vi "eyecat MAX v2-1_JS_160308.vi"() -> ()   [LabVIEW 2014]
doc: "This VI is an upgrade from the WIN 1_v4 that implements the ageing subrutine"
uses:
  Buttons/String output.ctl
  <vilib>/Utility/miscctls.llb/LVRowAndColumnTypeDef.ctl
  Buttons/Numeric control.ctl
  Buttons/String input.ctl
  Buttons/Numeric indicator.ctl
  Controls Win/Control 3.ctl
  <vilib>/Platform/TimedLoop/XDataNode/nitl_modes.ctl
  <vilib>/Platform/TimedLoop/XDataNode/timing_clust.ctl
  <vilib>/Platform/TimedLoop/XDataNode/wakeup.ctl
  <vilib>/Utility/file.llb/Write To Spreadsheet File (string).vi
  <vilib>/Utility/file.llb/Read From Spreadsheet File (string).vi
  <vilib>/Utility/file.llb/Read From Spreadsheet File (DBL).vi
  <vilib>/regexp/Match Regular Expression.xnode
  <vilib>/Platform/TimedLoop/XDataNode/XDataNode.xnode
  <vilib>/Platform/TimedLoop/XDataNode/XDNodeRunTimeDep.lvlib
panel:
  out "Mexa_One Emissions":dbl[](array[numeric])
  out "Advanced Logging":bool
  out "Full System":bool
  out "MKS":bool
  in  "Alarm":bool
  in  "Analyser":bool
  in  "MFC":bool
  in  "System":bool
  in  "Ageing":bool
  in  "Performance":bool
  in  "Home":bool
  out "NO":dbl[](array[numeric])
  out "CO":dbl[](array[numeric])
  out "Mexa One":bool
  out "Pressure":dbl
  in  "Duration -1":i32
  in  "Demo Sync":i32
  in  "Demo On":bool
  in  "FlowGuide":bool
  in  "Mean(Off)/Interval(On) 2":bool
  in  "Flow Band %":dbl=1.04
  in  "Flow Sync":i32
  out "Emissions":dbl[](array[numeric])
  in  "Temperature Sync":i32
  in  "TempGuide":bool
  in  "Temp Band %":dbl=1.04
  in  "Mean(Off)/Interval(On)":bool
  in  "MKS 5Hz":bool
  out "output cluster":T2
  out "Lambda":dbl[](array[numeric])
  out "MKS HC":dbl
  in  "HC Index":i32
  out "Open/Closed \nLoop":dbl[](array[numeric])
  out "Air Cyc 2":dbl[](array[numeric])
  in  "Cycle size":i32
  out "ExtAnDn":bool
  out "ExtAnUp":bool
  out "HC Cyc 2":dbl[](array[numeric])
  out "SO Valve 2":dbl[](array[numeric])
  out "SO Valve 1":dbl[](array[numeric])
  out "Air Bal":dbl[](array[numeric])
  out "HC Bal":dbl[](array[numeric])
  out "Air Cyc 1":dbl[](array[numeric])
  out "HC Cyc 1":dbl[](array[numeric])
  out "File name":string
  out "Log?":bool
  out "Connected":bool
  out "Furnace temp 2":dbl
  out "Log interval (seconds)":T1
  in  "Flow rate Age":dbl
  in  "Inlet temp Age":dbl
  out "Stopped?":bool
  in  "Stop Cmd":T1
  out "Connected?":bool
  out "Error":dbl
  out "Iteration Duration":i64
  out "Finished Late? [i-1]":bool
  out "Furnace temp 1":dbl
  out "stop 2":bool
  in  "Enum 1":i16=1
  in  "Acknowledge":bool
  out "Test number":u16
  out "Flag1":bool=TRUE
  out "EditPos Subc":T3
  out "Flag 2":bool=TRUE
  in  "Tab Control":T4(tab)
  out "Warm Up":bool
  in  "Leak Test":bool
  in  "Stop Test":bool
  in  "Log Test Data":bool
  in  "Start Test":bool
  in  "Adv Settings":bool
  out "Doors Unlocked":bool
  in  "Temperature Limit (°C)":T1=1200.0 min=0.0 max=1200.0 step=1.0
  in  "File Name":T5="Test"
  in  "File Path":path=path "C:/DATA LOG"
  out "Fail":bool
  out "Pass":bool
  in  "Select Test Type":T6(radio)
  out "Standby":bool
  out "Doors Open":bool
  out "Extractor Fan On":bool
  out "Test In Progress":bool
  out "Cool Down":bool
  out "System Alarm":bool
  in  "Inlet Temperature (°C)":T1=400.0 min=350.0 max=1000.0 step=1.0
  in  "Inlet LAMBDA Lean":T1=1.2 min=1.02 max=3.0 step=0.001
  in  "Test Stop temperature (°C)":T1=300.0 min=100.0 max=1000.0 step=1.0
  in  "Test Start Temperature (°C)":T1=125.0 min=0.0 max=500.0 step=1.0
  in  "Furnace Ramp Rate (°C/min)":T1=15.0 min=1.0 max=50.0 step=0.1
  in  "NO:CO Ratio":T1=1.1 min=1.0 max=5.0 step=0.1
  in  "Inlet O2 (%)":T1=0.5 min=0.0 max=14.0 step=0.01
  in  "Inlet LAMBDA":T1=1.0 min=0.6 max=3.0 step=0.001
  out "Space Velocity (h-1)":T7
  out "Vol Flow @ STP (l/min)":T7
  in  "Test Flow Rate(g/s)":T1 min=0.0 max=100.0 step=0.01
  out "Sample Volume (litres)":T7
  in  "Number of Samples":T1=1.0 min=1.0 max=6.0 step=1.0
  in  "Sample Diameter (mm)":T1
  out "CO Theory (%) NO":T7 format="%#_3g"
  out "CO Theory (%)":T7 format="%#_3g"
  out "HC Theory (%)":T7
  in  "Sample Length (mm)":T1 min=0.0 step=0.5
  in  "NO ppm SW":dbl=500.0 caption="NO (ppm)" min=0.0 max=500.0 step=1.0
  in  "NO ppm Loff":T1 caption="NO ppm"
  in  "Delete sCycle":bool
  in  "Load sCycle":bool
  in  "Save sCycle":bool
  in  "Clear subcycle":bool
  in  "Clear Cycle Pattern":bool
  in  "Save Cycle":bool
  in  "Load Cycle":bool
  in  "Delete Cycle":bool
  out "Test Compiled":bool
  in  "Compile Test Button":bool
  in  "Sub-Cycle List":i32(listbox)=1
  in  "Cycle List":i32(listbox)=2
  out "Total Test Duration (hrs)":T8
  in  "Ageing Gas":enum32{"Radio Selection 1", "Radio Selection 2"}(radio)
  in  "Sub-Cycle Pattern":string[][](table) caption="Subcycle pattern"
  in  "Total Number of Cycles":T1=1.0 min=1.0 max=10000.0 step=1.0
  in  "Cycle Pattern":string[][](table)
  in  "Sub-Cycle Name":T5
  in  "Cycle Name":T5
  out "Heat Exchanger Temperatures (°C)":dynamicdata(graph)
  out "Flow Rate (g/s)":dynamicdata(graph)
  out "Sample Temperatures (°C)":dynamicdata(graph)
  out "System Temperatures (°C)":dynamicdata(graph)
  in  "Graph 1 Box":string(combo)="CO"
  in  "Graph 4 Box":string(combo)="NO"
  in  "Graph 3 Box":string(combo)="Air Cycle 1"
  in  "Graph 2 Box":string(combo)="HC Cycle 1"
  out "MFC Graph 4":dynamicdata(graph)
  out "MFC Graph 3":dynamicdata(graph)
  out "MFC Graph 1":dynamicdata(graph)
  out "MFC Graph 2":dynamicdata(graph)
  out "HC Concentration (ppm)":dynamicdata(graph)
  out "Lambda":dynamicdata(graph)
  out "O2/CO Concentration":dynamicdata(graph)
  out "NO Concentration (ppm)":dynamicdata(graph)
  in  "Purge System":bool
  in  "Alarm ack":bool
  in  "Clear log":bool
  out "Table":string[][](table)
  out "Soft Alarm":bool
  out "Hard Alarm":bool
  # "1% = 0.01"
  # "Test Type"
  # "Test Commands"
  # "System Indicators"
  # "Leak Test"
  # "Catalyst Specification"
  # "Lightoff Settings"
  # "Furnace Lightoff Settings"
  # "Sweep Settings"
  # "CO/HC Lightoff Settings"
  # "0.96 < lambda < 0.85"
  # "1.02< lambda < 1.6"
  # "350 < Tinlet < 1000"
  # "NO Lightoff Settings"
  # "Flow Specification"
  # "Cycle Compiled"
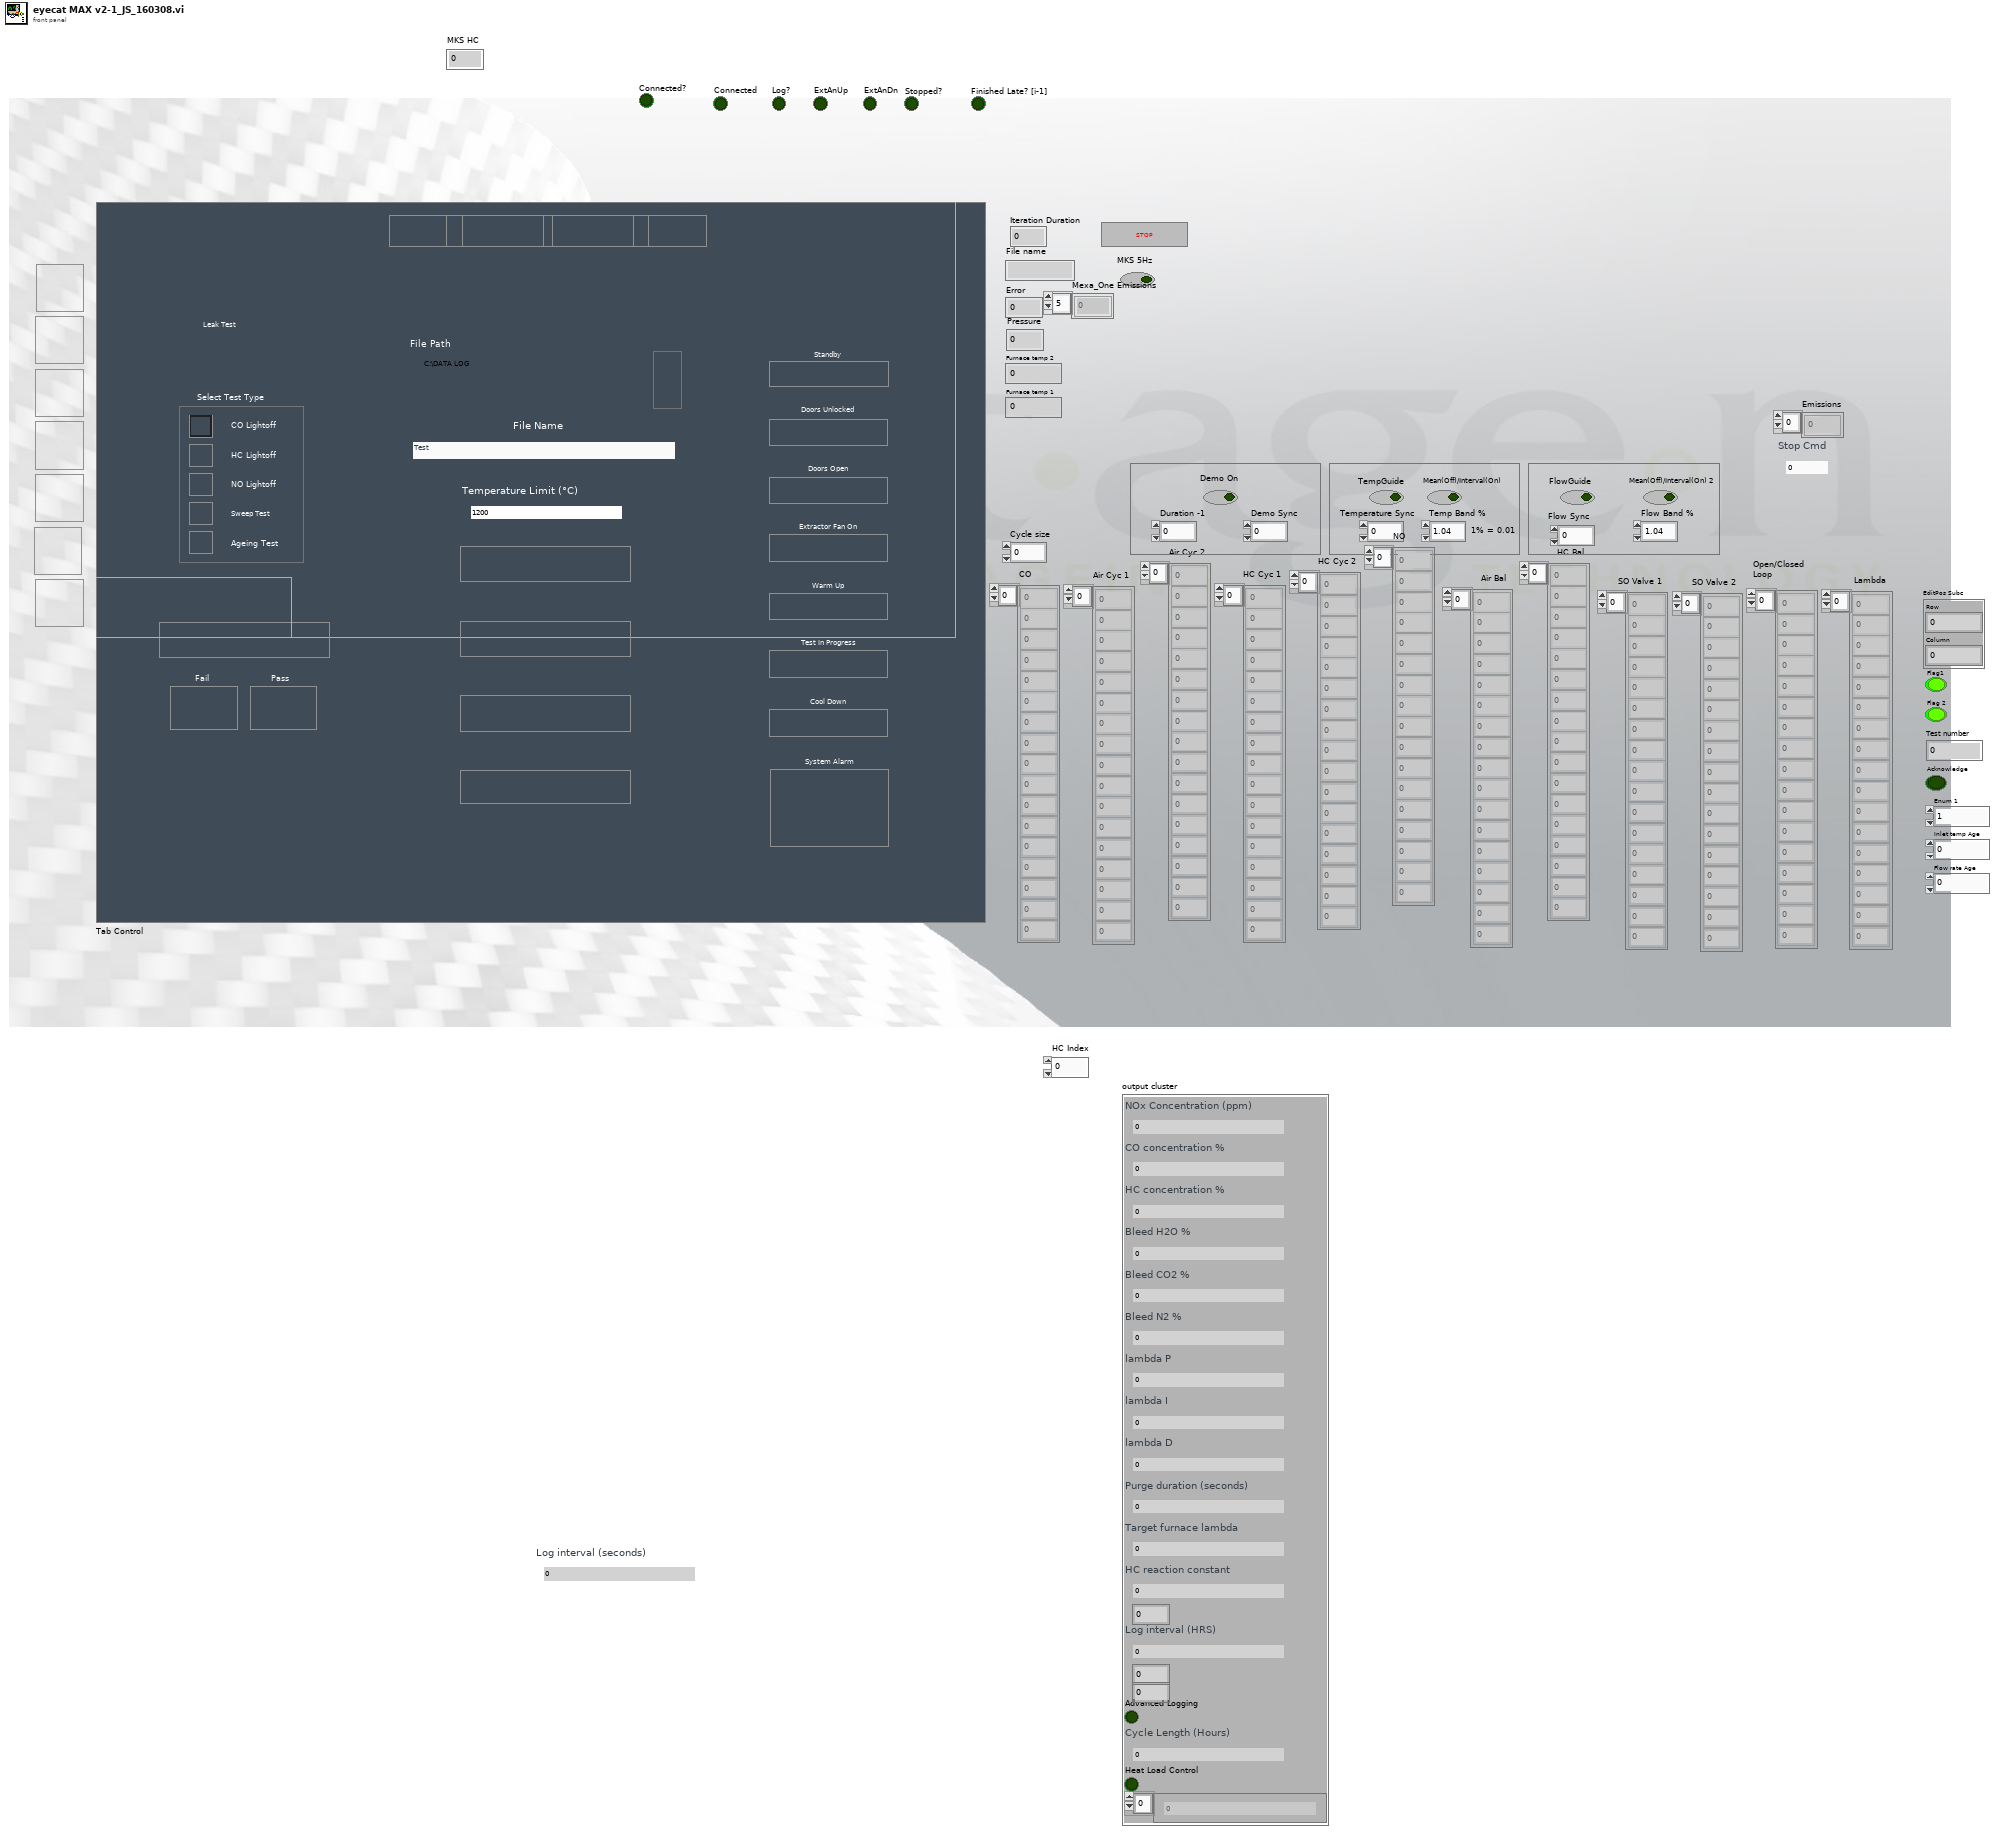
[diagram p1: front panel]
types:
  T1 = typedef "Numeric control.ctl" = dbl
  T2 = cluster{"NOx Concentration (ppm)":T1, "CO concentration %":T1, "HC concentration %":T1, "Bleed H2O %":T1, "Bleed CO2 %":T1, "Bleed N2 %":T1, "lambda P":T1, "lambda I":T1, "lambda D":T1, "Purge duration (seconds)":T1, "Target furnace lambda":T1, "HC reaction constant":T1, i16, "Log interval (HRS)":T1, i16, i16, "Advanced Logging":bool, "Cycle Length (Hours)":T1, "Heat Load Control":bool, T1[]}
  T3 = typedef "LVRowAndColumnTypeDef.ctl" = cluster{"Row":i32, "Column":i32}
  T4 = enum32{"MAIN", "PERFORMANCE TEST SETUP", "AGEING TEST SETUP", "SYSTEM DATA", "MFC", "ANALYSER DATA", "ALARM LOG"}
  T5 = typedef "String input.ctl" = string
  T6 = enum32{"CO Lightoff", "HC Lightoff", "NO Lightoff", "Sweep Test", "Ageing Test"}
  T7 = typedef "Numeric indicator.ctl" = dbl
  T8 = typedef "String output.ctl" = string
  T9 = typedef "XDNodeRunTimeDep.lvlib/nitl_modes.ctl" = enum32{"No Change", "Process missed periods, maintain original phase", "Discard missed periods, maintain original phase", "Process missed periods, ignore original phase", "Discard missed periods, ignore original phase"}
  T10 = typedef "Control 3.ctl" = enum16{"main", "start test", "save subc", "load subc", "delete subc", "clear table 1", "update list 1", "save cycle", "load cycle", "delete cycle", "clear table 2", "update list 2", "calc HC CO", "Total time calc", "update Cycle pattern ", "load cycle name", "convert to num", "load test array", "check scycle name", "check cycle name", "Multigas connect", "Multigas disconnect", "Leak Test", "Import Cycle", "Display Graph"}
  T11 = enum8{"Enabled", "Disabled", "Disabled and Grayed Out"}
  T12 = typedef "XDNodeRunTimeDep.lvlib/timing_clust.ctl" = cluster{"Expected End [f-1]":u64, "Actual End [f-1]":u64, "Finished Late? [f-1]":bool, "Expected End [i-1]":u64, "Actual End [i-1]":u64, "Finished Late? [i-1]":bool, "Expected Start [i]":u64, "Actual Start [i]":u64, "Expected Start [f]":u64, "Actual Start [f]":u64, "Source Name":string, "Structure Name":string, "Period":i64, "Deadline":i64, "Offset":i64, "Start":i64, "Priority":i32, "Timeout":i32, "Mode":T9, "Wakeup Reason":T13, "Error":errorcluster, "Source Type":string, "Secondary Source Type":string, "Global End Time":u64, "Global Start Time":u64, "Frame Duration":u64, "Iteration Duration":u64, "Assigned CPU":i32, "I/O Scan Engine Mode":u32}
  T13 = typedef "XDNodeRunTimeDep.lvlib/wakeup.ctl" = enum32{"Normal", "Aborted", "Asynchronous wakeup", "Timing source error", "Timed loop error", "Timeout"}
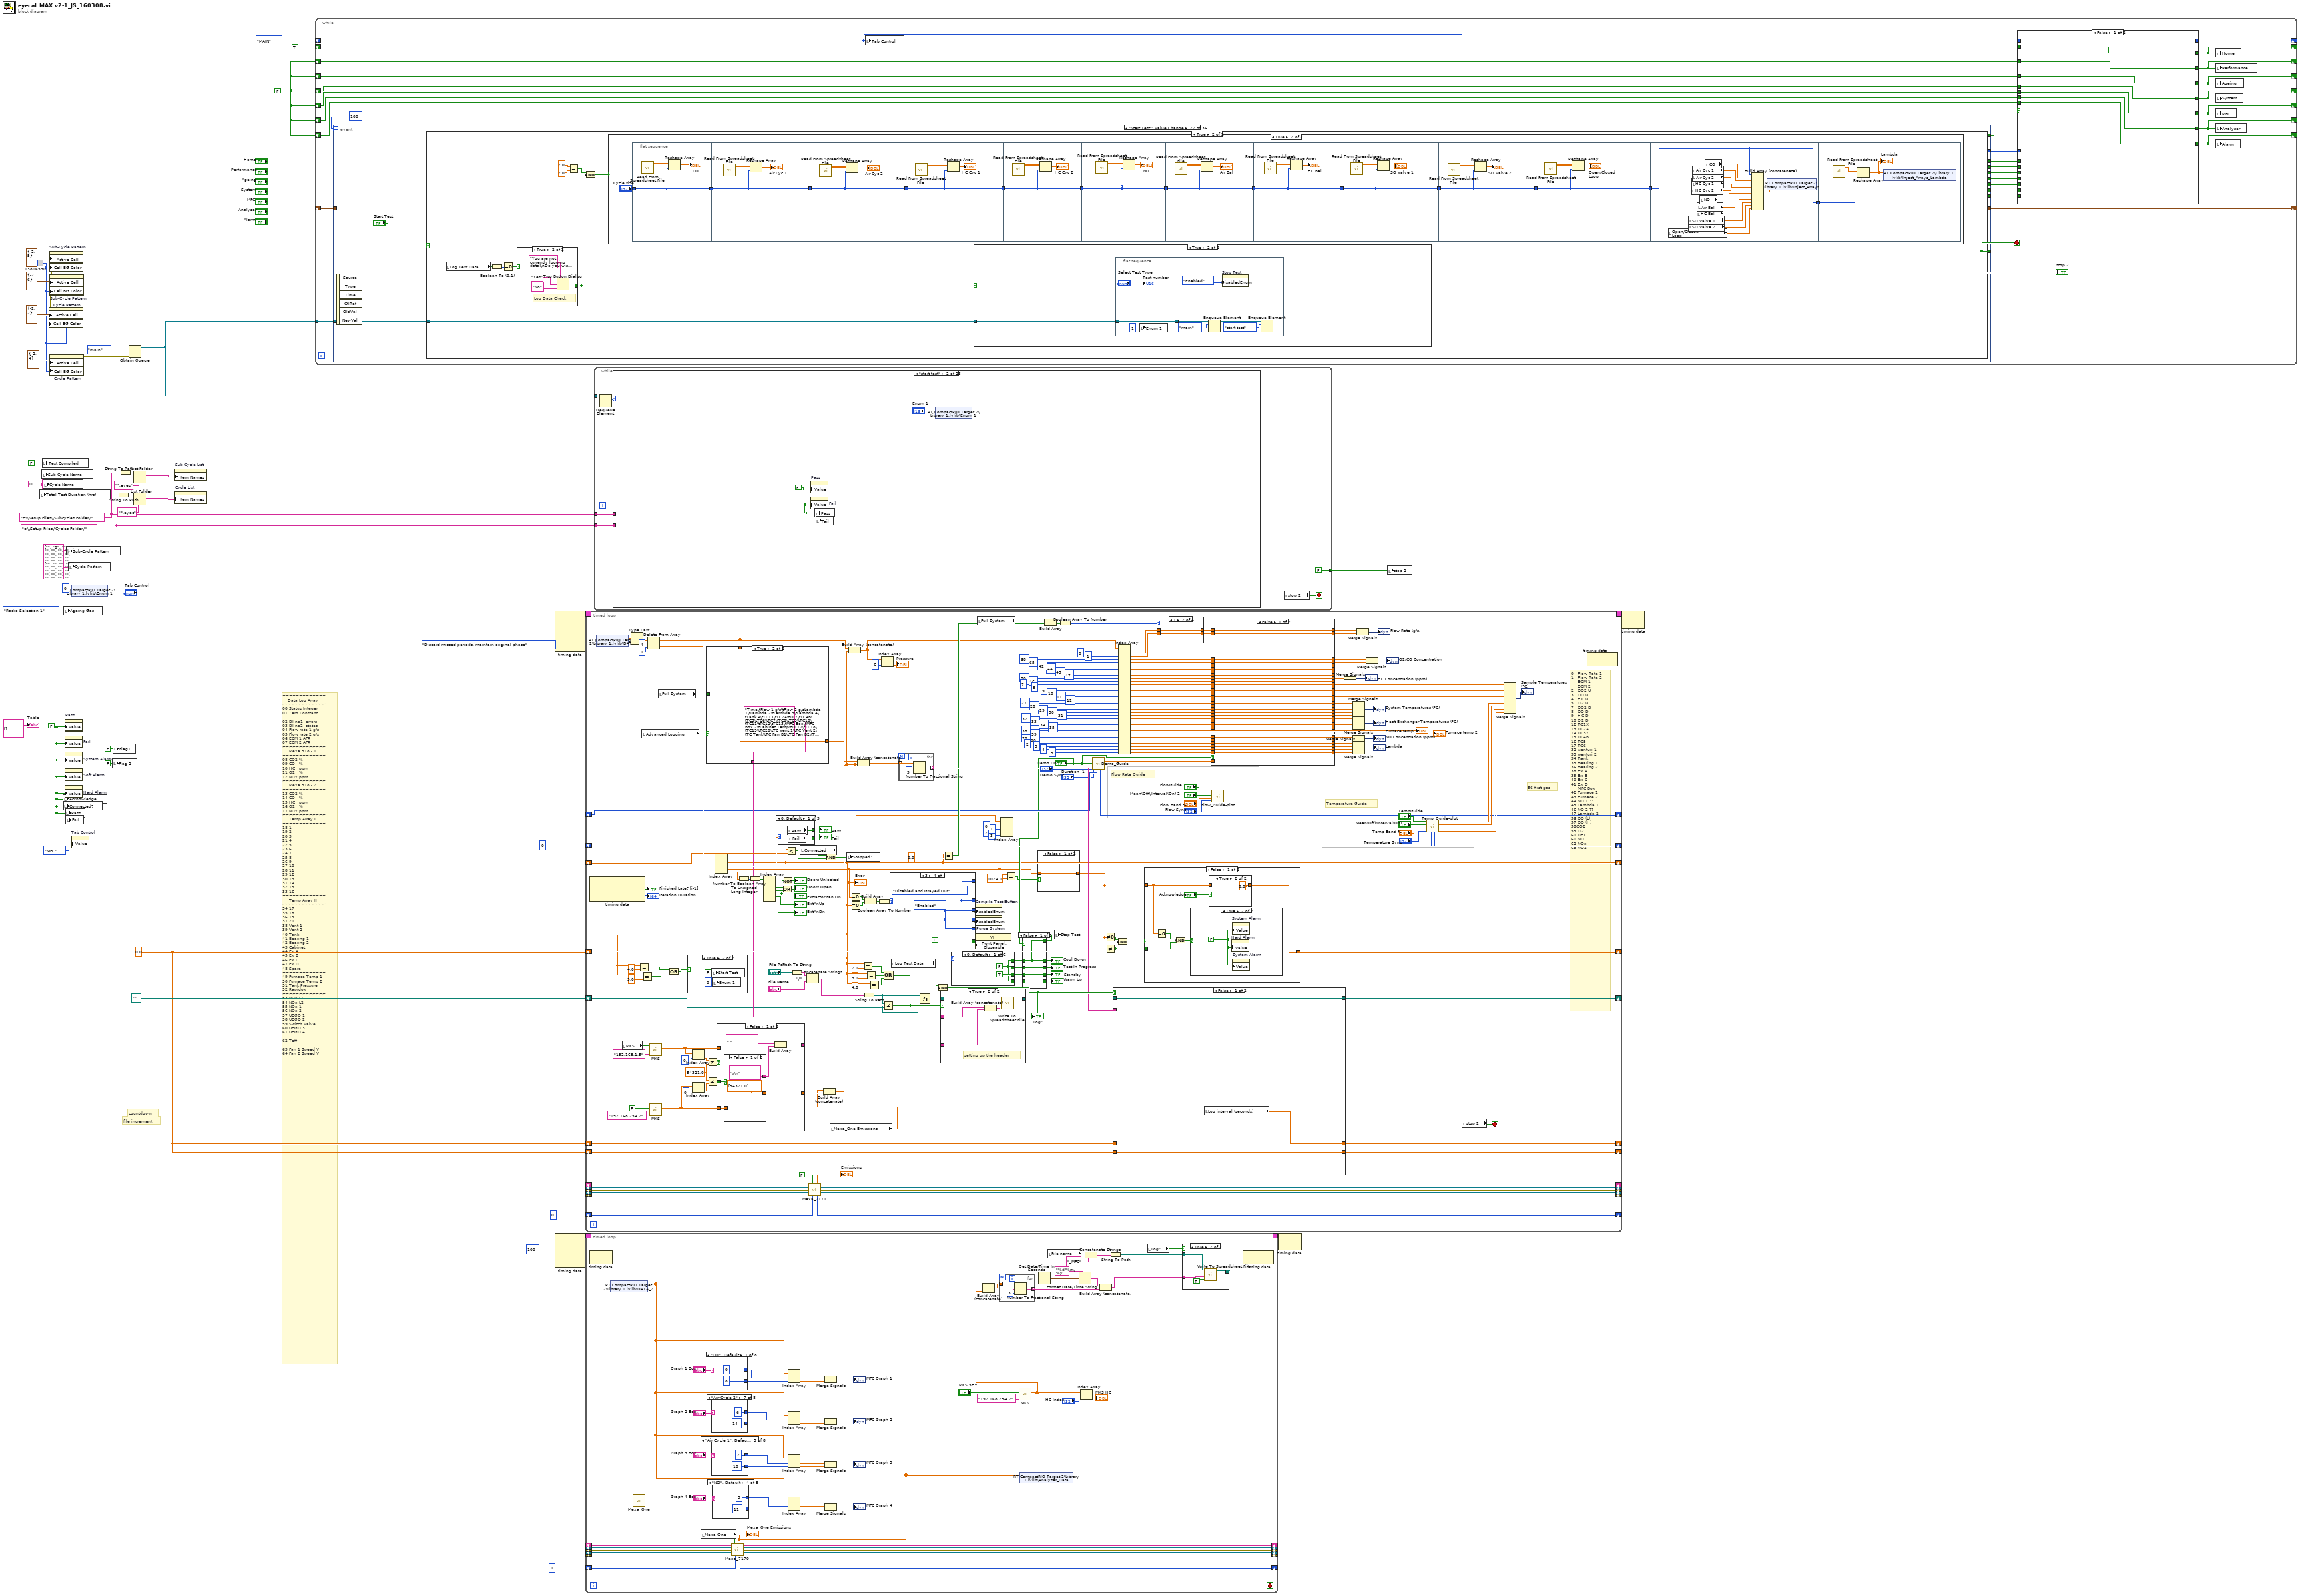
[diagram p0: block diagram]
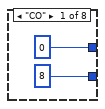
[diagram p2: hidden frame]
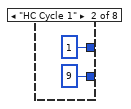
[diagram p3: hidden frame]
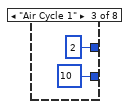
[diagram p4: hidden frame]
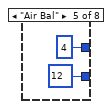
[diagram p5: hidden frame]
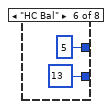
[diagram p6: hidden frame]
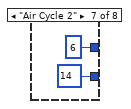
[diagram p7: hidden frame]
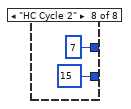
[diagram p8: hidden frame]
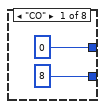
[diagram p9: hidden frame]
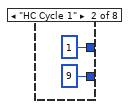
[diagram p10: hidden frame]
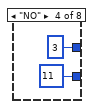
[diagram p11: hidden frame]
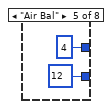
[diagram p12: hidden frame]
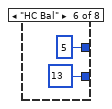
[diagram p13: hidden frame]
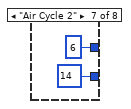
[diagram p14: hidden frame]
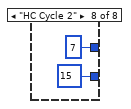
[diagram p15: hidden frame]
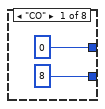
[diagram p16: hidden frame]
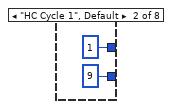
[diagram p17: hidden frame]
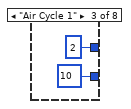
[diagram p18: hidden frame]
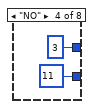
[diagram p19: hidden frame]
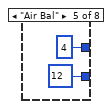
[diagram p20: hidden frame]
diagram:
  (unwired) 0 ("index")
  w2 = FALSE
  (unwired) 0 ("index")
  w10 = FALSE
  w9 = 0.0 ("y")
  w25 = ""
  w28 = "c:\\Setup Files\\Cycles Folder\\"
  w34 = u32 13816530
  w26 = "c:\\Setup Files\\Subcycles Folder\\"
  # "~~~~~~~~~~~~~\n    Data Log Array\n~~~~~~~~~~~~~\n00 Status Integer\n01 Zero Constant\n\n02 DI no1 -errors\n03 DI no2 -states\n04 Flow rate 1 g/s\n05 Flow rate 2 g/s\n06 ECM 1 AFR\n07 ECM 2 AFR\n~~~~~~~~~~~~~\n     Mexa 518 - 1\n~~~~~~~~~~~~~\n08 CO2 %\n09 CO   %\n10 HC   ppm\n11 O2   %\n12 NOx ppm\n~~~~~~~~~~~~~\n     Mexa 518 - 2\n~~~~~~~~~~~~~\n13 CO2 %\n14 CO   %\n15 HC   ppm\n16 O2   %\n17 NOx ppm\n~~~~~~~~~~~~~\n     Temp Array I\n~~~~~~~~~~~~~\n18 1\n19 2 \n20 3\n21 4\n22 5\n23 6\n24 7\n25 8\n26 9\n27 10\n28 11\n29 12\n30 13\n31 14\n32 15\n33 16\n~~~~~~~~~~~~~\n     Temp Array II\n~~~~~~~~~~~~~\n34 17\n35 18\n36 19\n37 20\n38 Vent 1\n39 Vent 2\n40 Tank\n41 Bearing 1\n42 Bearing 2\n43 Cabinet\n44 Ex A\n45 Ex B\n46 Ex C\n47 Ex D\n48 Spare\n~~~~~~~~~~~~~\n49 Furnace Temp 1\n50 Furnace Temp 2\n51 Tank Pressure\n52 Rapidox\n~~~~~~~~~~~~~\n53 NOx L1\n54 NOx L2\n55 NOx 1\n56 NOx 2\n57 UEGO 1\n58 UEGO 2\n59 Switch Valve\n60 UEGO 3\n61 UEGO 4\n\n62 Teff\n\n63 Fan 1 Speed V\n64 Fan 2 Speed V"
  # "file increment"
  # "countdown"
  n1 = local write "Total Test Duration (hrs)"(w25) -> ()
  n2 = local write "Sub-Cycle Name"(w25) -> ()
  n3 = local write "Test Compiled"(FALSE ("Cycle Compiled")) -> ()
  n4 = local write "Cycle Name"(w25) -> ()
  n5 = property on="Sub-Cycle Pattern" class="Tbl (strict)"("Active Cell"=T3 {"Row"=-2, "Column"=5} ("Active Cell:Active Cell"), "Cell BG Color"=w34) -> (error out=w39:errorcluster)  [unwired: 2 in, 1 out]
  n6 = property on="Sub-Cycle Pattern" class="Tbl (strict)"(error in=w39, "Active Cell"=T3 {"Row"=-2, "Column"=6} ("Active Cell:Active Cell"), "Cell BG Color"=w34) -> (error out=w38:errorcluster)  [unwired: 1 in, 1 out]
  n7 = property on="Cycle Pattern" class="Tbl (strict)"(error in=w38, "Active Cell"=T3 {"Row"=-2, "Column"=2} ("Active Cell:Active Cell"), "Cell BG Color"=w34) -> (error out=w36:errorcluster)  [unwired: 1 in, 1 out]
  n8 = property on="Cycle Pattern" class="Tbl (strict)"(error in=w36, "Active Cell"=T3 {"Row"=-2, "Column"=4} ("Active Cell:Active Cell"), "Cell BG Color"=w34) -> (error out=w33:errorcluster)  [unwired: 1 in, 1 out]
  n9 = local write "Acknowledge"(w10) -> ()
  n10 = local write "Connected?"(w10) -> ()
  n11 = local write "Ageing Gas"(enum32{"Radio Selection 1", "Radio Selection 2"}."Radio Selection 1" ("Ageing Gas")) -> ()
  n12 = property on="Pass" class="Bool (strict)"("Value"=w10) -> ()  [unwired: 2 in, 2 out]
  n13 = property on="Fail" class="Bool (strict)"("Value"=w10) -> ()  [unwired: 2 in, 2 out]
  n14 = property on="System Alarm" class="Bool (strict)"("Value"=w10) -> ()  [unwired: 2 in, 2 out]
  n15 = property on="Soft Alarm" class="Bool (strict)"("Value"=w10) -> ()  [unwired: 2 in, 2 out]
  n16 = property on="Hard Alarm" class="Bool (strict)"("Value"=w10) -> ()  [unwired: 2 in, 2 out]
  n17 = local write "Pass"(w10) -> ()
  n18 = local write "Fail"(w10) -> ()
  n19 = local write "Sub-Cycle Pattern"(string[][] [["", "0", "", "", "", "", "", "", "", "", "", "", ""], ["", "", "", "", "", "", "", "", "", "", "", "", ""], ["", "", "", "", "", "", "", "", "", "", "", "", ""], ["", "", "", "", "", "", "", "", "", "", "", "", ""], ["", "", "", "", "", "", "", "", "", "", "", "", ""], ["", "", "", "", "", "", "", "", "", "", "", "", ""], ["", "", "", "", "", "", "", "", "", "", "", "", ""], ["", "", "", "", "", "", "", "", "", "", "", "", ""], ["", "", "", "", "", "", "", "", "", "", "", "", ""], ["", "", "", "", "", "", "", "", "", "", "", "", ""], ["", "", "", "", "", "", "", "", "", "", "", "", ""], ["", "", "", "", "", "", "", "", "", "", "", "", ""], ["", "", "", "", "", "", "", "", "", "", "", "", ""], ["", "", "", "", "", "", "", "", "", "", "", "", ""], ["", "", "", "", "", "", "", "", "", "", "", "", ""], ["", "", "", "", "", "", "", "", "", "", "", "", ""], ["", "", "", "", "", "", "", "", "", "", "", "", ""], ["", "", "", "", "", "", "", "", "", "", "", "", ""], ["", "", "", "", "", "", "", "", "", "", "", "", ""], ["", "", "", "", "", "", "", "", "", "", "", "", ""], ["", "", "", "", "", "", "", "", "", "", "", "", ""], ["", "", "", "", "", "", "", "", "", "", "", "", ""], ["", "", "", "", "", "", "", "", "", "", "", "", ""], ["", "", "", "", "", "", "", "", "", "", "", "", ""], ["", "", "", "", "", "", "", "", "", "", "", "", ""], ["", "", "", "", "", "", "", "", "", "", "", "", ""], ["", "", "", "", "", "", "", "", "", "", "", "", ""], ["", "", "", "", "", "", "", "", "", "", "", "", ""], ["", "", "", "", "", "", "", "", "", "", "", "", ""], ["", "", "", "", "", "", "", "", "", "", "", "", ""], ["", "", "", "", "", "", "", "", "", "", "", "", ""]]) -> ()
  n20 = local write "Cycle Pattern"(string[][] [["", "", "", "", ""], ["", "", "", "", ""], ["", "", "", "", ""], ["", "", "", "", ""], ["", "", "", "", ""], ["", "", "", "", ""], ["", "", "", "", ""], ["", "", "", "", ""], ["", "", "", "", ""], ["", "", "", "", ""], ["", "", "", "", ""], ["", "", "", "", ""], ["", "", "", "", ""], ["", "", "", "", ""], ["", "", "", "", ""], ["", "", "", "", ""], ["", "", "", "", ""], ["", "", "", "", ""], ["", "", "", "", ""], ["", "", "", "", ""], ["", "", "", "", ""], ["", "", "", "", ""], ["", "", "", "", ""], ["", "", "", "", ""], ["", "", "", "", ""], ["", "", "", "", ""], ["", "", "", "", ""], ["", "", "", "", ""], ["", "", "", "", ""], ["", "", "", "", ""], ["", "", "", "", ""]]) -> ()
  n21 = shared-variable "RT CompactRIO Target 2\\Library 1.lvlib\\Enum 1"(u16 0 ("Enum 1")) -> ()  [unwired: 1 in, 1 out]
  n22 = property on="Tab Control" class="TabCtl (strict)"("Value"=T4."MFC" ("Tab Control")) -> ()  [unwired: 2 in, 2 out]
  n23 = local write "Flag 2"(FALSE) -> ()
  n24 = local write "Flag1"(FALSE) -> ()
  n25 = String To Path(string=w28) -> (path=w29:path)
  n26 = String To Path(string=w26) -> (path=w31:path)
  n27 = Obtain Queue(element data type=Control_3."main" ("Enum"), error in (no error)=w33) -> (queue out=w42:refnum<queue>)  [unwired: 3 in, 2 out]
  n28 = List Folder(path=w29, pattern="*.eyec") -> (filenames=w30:string[])  [unwired: 2 in, 3 out]
  n29 = List Folder(path=w31, pattern="*.eyes") -> (filenames=w32:string[])  [unwired: 2 in, 3 out]
  n30 = property on="Sub-Cycle List" class="LstBox (strict)"("Item Names"=w32) -> ()  [unwired: 2 in, 2 out]
  n31 = property on="Cycle List" class="LstBox (strict)"("Item Names"=w30) -> ()  [unwired: 2 in, 2 out]
  n32 = while {
    tunnel: w42 -> [w73]
    shift-right: [w71] -> _
    shift-left: _ -> [w70]
    shift-right: [w68] -> _
    shift-left: T4."MAIN" ("Tab Control") -> [w67]
    shift-right: [w56] -> _
    shift-left: w2 -> [w49]
    shift-right: [w57] -> _
    shift-left: TRUE -> [w50]
    shift-right: [w55] -> _
    shift-left: w2 -> [w44]
    shift-right: [w54] -> _
    shift-left: w2 -> [w45]
    shift-right: [w53] -> _
    shift-left: w2 -> [w46]
    shift-right: [w52] -> _
    shift-left: w2 -> [w47]
    shift-right: [w51] -> _
    shift-left: w2 -> [w48]
    stop <- w69 stop-if-true
    n33 = event shown="[21] \"Start Test\": Value Change" {
      selector: _ -> [_ _ _ _ _ _ _ _ _ _ _ _ _ _ _ _ _ _ _ _ _ _ _ _ _ _ _ _ _ _ _ _ _ _ _ _]
      dyn-events: _ -> [_ _ _ _ _ _ _ _ _ _ _ _ _ _ _ _ _ _ _ _ _ _ _ _ _ _ _ _ _ _ _ _ _ _ _ _]
      timeout: 100 -> [_ _ _ _ _ _ _ _ _ _ _ _ _ _ _ _ _ _ _ _ _ _ _ _ _ _ _ _ _ _ _ _ _ _ _ _]
      tunnel: w73 -> [w92 w94 _ w103 w111 w118 w125 w136 w140 w151 w156 w159 w164 w186 w194 w195 _ _ _ _ w239 w250 _ w342 w366 _ w380 _ _ _ _ _ _ _ _ _]
      tunnel: [w90 w93 _ w104 w110 w117 w124 w135 w138 w146 w153 w158 w162 w183 _ _ _ _ _ _ _ _ _ _ _ _ _ _ _ _ _ _ _ _ _ _] -> w71
      tunnel: w70 -> [w90 w93 _ w104 w110 w117 w123 w135 w138 w146 w153 w158 w162 w183 _ _ _ _ _ _ _ _ _ _ _ _ _ _ _ _ _ _ _ _ _ _]
      tunnel: [_ _ w96 _ _ _ _ _ _ _ _ _ _ _ _ _ _ _ _ _ _ _ _ _ _ _ _ _ _ _ _ _ _ _ _ _] -> w69
      tunnel: [_ _ _ _ _ _ _ _ _ _ _ _ _ _ _ _ _ _ _ _ _ _ _ _ _ _ _ _ _ TRUE TRUE TRUE TRUE TRUE TRUE TRUE] -> w66
      tunnel: [_ _ _ _ _ _ _ _ _ _ _ _ _ _ _ _ _ _ _ _ _ _ _ _ _ _ _ _ _ T4."MAIN" ("Tab Control") T4."PERFORMANCE TEST SETUP" ("Tab Control") T4."AGEING TEST SETUP" ("Tab Control") T4."SYSTEM DATA" ("Tab Control") T4."MFC" ("Tab Control") T4."ANALYSER DATA" ("Tab Control") T4."ALARM LOG" ("Tab Control")] -> w65
      tunnel: [_ _ _ _ _ _ _ _ _ _ _ _ _ _ _ _ _ _ _ _ _ _ _ _ _ _ _ _ _ TRUE w391 w395 w399 w403 w408 w411] -> w64
      tunnel: [_ _ _ _ _ _ _ _ _ _ _ _ _ _ _ _ _ _ _ _ _ _ _ _ _ _ _ _ _ w388 TRUE w395 w399 w403 w408 w411] -> w63
      tunnel: [_ _ _ _ _ _ _ _ _ _ _ _ _ _ _ _ _ _ _ _ _ _ _ _ _ _ _ _ _ w388 w391 TRUE w399 w403 w408 w411] -> w62
      tunnel: [_ _ _ _ _ _ _ _ _ _ _ _ _ _ _ _ _ _ _ _ _ _ _ _ _ _ _ _ _ w388 w391 w395 TRUE w403 w408 w411] -> w61
      tunnel: [_ _ _ _ _ _ _ _ _ _ _ _ _ _ _ _ _ _ _ _ _ _ _ _ _ _ _ _ _ w388 w391 w395 w399 TRUE w408 w411] -> w60
      tunnel: [_ _ _ _ _ _ _ _ _ _ _ _ _ _ _ _ _ _ _ _ _ _ _ _ _ _ _ _ _ w388 w391 w395 w399 w403 TRUE w411] -> w59
      tunnel: [_ _ _ _ _ _ _ _ _ _ _ _ _ _ _ _ _ _ _ _ _ _ _ _ _ _ _ _ _ w388 w391 w395 w399 w403 w408 TRUE] -> w58
      event Timeout {
        n34 = event-data() -> ()  [unwired: 1 in, 2 out]
        n35 = Enqueue Element(queue=w92, element=Control_3."main" ("Enum")) -> ()  [unwired: 2 in, 3 out]
      }
      event "Clear subcycle": Value Change {
        n36 = event-data() -> ()  [unwired: 1 in, 5 out]
        n37 = Enqueue Element(queue=w94, element=Control_3."clear table 1" ("Enum")) -> ()  [unwired: 2 in, 3 out]
      }
      event Panel Close? {
        n38 = event-data() -> ()  [unwired: 1 in, 3 out]
        n39 = Two Button Dialog(message="This command will close Eyecat!\nDo you wish to continue?", 1:"No" ("F button name (\"Cancel\")"), 2:"Yes" ("T button name (\"OK\")")) -> (T button?=w96:bool)
        n40 = Not(x=w96) -> (.not. x?=w97:bool)
        n41 = event-data("Discard?"=w97) -> ()  [unwired: 1 in, 1 out]
      }
      event "Save sCycle": Value Change {
        n42 = event-data() -> ()  [unwired: 1 in, 5 out]
        n43 = local read "Sub-Cycle Pattern"() -> (w101:string[][])
        n44 = call "Time column check.vi"("Array"=w101) -> ("Mistake?"=w102:bool)  [unwired: 10 in]
        n45 = case shown="False" w102 {
          tunnel: w103 -> [w105 _]
          frame False {
            n46 = Enqueue Element(queue=w105, element=Control_3."save subc") -> (queue out=w107:refnum<queue>)  [unwired: 2 in, 2 out]
            n47 = Enqueue Element(queue=w107, element=Control_3."update list 1") -> ()  [unwired: 2 in, 3 out]
          }
          frame True {
            n48 = One Button Dialog(message="The time sequence is incorrect!\nReview and save again!") -> ()  [unwired: 1 in, 1 out]
          }
        }
      }
      event "Load sCycle": Value Change {
        n49 = event-data() -> ()  [unwired: 1 in, 5 out]
        n50 = Enqueue Element(queue=w111, element=Control_3."load subc") -> ()  [unwired: 2 in, 3 out]
      }
      event "Delete sCycle": Value Change {
        n51 = event-data() -> ()  [unwired: 1 in, 5 out]
        n52 = Enqueue Element(queue=w118, element=Control_3."delete subc") -> (queue out=w120:refnum<queue>)  [unwired: 2 in, 2 out]
        n53 = Enqueue Element(queue=w120, element=Control_3."update list 1") -> (queue out=w116:refnum<queue>)  [unwired: 2 in, 2 out]
        n54 = Enqueue Element(queue=w116, element=Control_3."update Cycle pattern ") -> (queue out=w113:refnum<queue>)  [unwired: 2 in, 2 out]
        n55 = Enqueue Element(queue=w113, element=Control_3."Total time calc") -> ()  [unwired: 2 in, 3 out]
      }
      event "Sub-Cycle Pattern": Mouse Down; "Sub-Cycle Pattern": Value Change {
        n56 = event-data() -> ()  [unwired: 1 in, 3 out]
        n57 = property on="Sub-Cycle Pattern" class="Tbl (strict)"() -> ("EditPos"=w124:T3)  [unwired: 2 in, 2 out]
        n58 = Unbundle By Name(w124) -> ("Row"=w126:i32)  [unwired: 1 out]
        n59 = Less?(x=w126, y=30) -> (x < y?=w128:bool)
        n60 = case shown="True" w128 {
          tunnel: w125 -> [_ w133]
          frame False {
            n61 = One Button Dialog(message="This table is limited to 30 entries!") -> ()  [unwired: 1 in, 1 out]
          }
          frame True {
            n62 = Enqueue Element(queue=w133, element=Control_3."convert to num") -> (queue out=w132:refnum<queue>)  [unwired: 2 in, 2 out]
            n63 = Enqueue Element(queue=w132, element=Control_3."calc HC CO") -> ()  [unwired: 2 in, 3 out]
          }
        }
        "EditPos Subc" <- w123
        "Flag1" <- TRUE
      }
      event "Clear Cycle Pattern": Value Change {
        n64 = event-data() -> ()  [unwired: 1 in, 5 out]
        n65 = Enqueue Element(queue=w136, element=Control_3."clear table 2" ("Enum")) -> ()  [unwired: 2 in, 3 out]
        n66 = local write "Test Compiled"(FALSE ("Test Compiled")) -> ()
      }
      event "Save Cycle": Value Change {
        n67 = event-data() -> ()  [unwired: 1 in, 5 out]
        n68 = Enqueue Element(queue=w140, element=Control_3."update Cycle pattern ") -> (queue out=w139:refnum<queue>)  [unwired: 2 in, 2 out]
        n69 = Enqueue Element(queue=w139, element=Control_3."save cycle") -> (queue out=w143:refnum<queue>)  [unwired: 2 in, 2 out]
        n70 = Enqueue Element(queue=w143, element=Control_3."update list 2") -> ()  [unwired: 2 in, 3 out]
      }
      event "Load Cycle": Value Change {
        n71 = event-data() -> ()  [unwired: 1 in, 5 out]
        n72 = Enqueue Element(queue=w151, element=Control_3."load cycle") -> (queue out=w149:refnum<queue>)  [unwired: 2 in, 2 out]
        n73 = Enqueue Element(queue=w149, element=Control_3."update Cycle pattern ") -> (queue out=w148:refnum<queue>)  [unwired: 2 in, 2 out]
        n74 = local write "Test Compiled"(FALSE ("Test Compiled")) -> ()
        n75 = Enqueue Element(queue=w148, element=Control_3."Total time calc") -> ()  [unwired: 2 in, 3 out]
      }
      event "Delete Cycle": Value Change {
        n76 = event-data() -> ()  [unwired: 1 in, 5 out]
        n77 = Enqueue Element(queue=w156, element=Control_3."delete cycle") -> (queue out=w155:refnum<queue>)  [unwired: 2 in, 2 out]
        n78 = Enqueue Element(queue=w155, element=Control_3."update list 2") -> ()  [unwired: 2 in, 3 out]
      }
      event Value Change {
        n79 = event-data() -> ()  [unwired: 1 in, 5 out]
        n80 = Enqueue Element(queue=w159, element=Control_3."Total time calc") -> ()  [unwired: 2 in, 3 out]
      }
      event "Cycle Pattern": Mouse Up; "Cycle Pattern": Value Change {
        n81 = event-data() -> ()  [unwired: 1 in, 3 out]
        n82 = property on="Cycle Pattern" class="Tbl (strict)"() -> ("EditPos"=w166:T3)  [unwired: 2 in, 2 out]
        n83 = Unbundle By Name(w166) -> ("Row"=w163:i32, "Column"=w168:i32)
        n84 = Less?(x=w163, y=30) -> (x < y?=w167:bool)
        n85 = case shown="True" w167 {
          tunnel: w168 -> [_ w170]
          tunnel: w164 -> [_ w173]
          frame False {
            n86 = One Button Dialog(message="This table is limited to 30 entries!") -> ()  [unwired: 1 in, 1 out]
          }
          frame True {
            n87 = Equal?(x=w170, y=1) -> (x = y?=w174:bool)
            n88 = case shown="True" w174 {
              tunnel: w173 -> [w177 w180]
              tunnel: [w176 w179] -> w172
              frame False {
                n89 = Enqueue Element(queue=w177, element=Control_3."update Cycle pattern ") -> (queue out=w176:refnum<queue>)  [unwired: 2 in, 2 out]
              }
              frame True {
                n90 = Enqueue Element(queue=w180, element=Control_3."load cycle name") -> (queue out=w179:refnum<queue>)  [unwired: 2 in, 2 out]
              }
            }
            n91 = Enqueue Element(queue=w172, element=Control_3."Total time calc") -> ()  [unwired: 2 in, 3 out]
          }
        }
        "Flag 2" <- TRUE
      }
      event "Compile Test Button": Value Change {
        n92 = event-data() -> ()  [unwired: 1 in, 5 out]
        n93 = local read "Flag 2"() -> (w182:bool)
        n94 = case shown="True" w182 {
          tunnel: w186 -> [w187 w191]
          tunnel: [w187 w188] -> w184
          frame False {
          }
          frame True {
            n95 = Enqueue Element(queue=w191, element=Control_3."save cycle") -> (queue out=w189:refnum<queue>)  [unwired: 2 in, 2 out]
            n96 = Enqueue Element(queue=w189, element=Control_3."update list 2") -> (queue out=w188:refnum<queue>)  [unwired: 2 in, 2 out]
          }
        }
        n97 = Enqueue Element(queue=w184, element=Control_3."load test array") -> ()  [unwired: 2 in, 3 out]
      }
      event Value Change {
        n98 = event-data() -> ()  [unwired: 1 in, 5 out]
        n99 = Enqueue Element(queue=w194, element=Control_3."check scycle name") -> ()  [unwired: 2 in, 3 out]
      }
      event Value Change {
        n100 = event-data() -> ()  [unwired: 1 in, 5 out]
        n101 = Enqueue Element(queue=w195, element=Control_3."check cycle name") -> ()  [unwired: 2 in, 3 out]
      }
      event Value Change {
        n102 = event-data() -> ()  [unwired: 1 in, 5 out]
        n103 = Square(x="Sample Diameter (mm)") -> (x^2=w204:T1)
        n104 = Compound Arithmetic op=MULTIPLY(w204, "Sample Length (mm)", "Number of Samples", 3.141592653589793) -> (w203:T1)
        n105 = Divide(x=w203, y=4000000.0) -> (x/y=→"Sample Volume (litres)":T1)
      }
      event Value Change {
        # "O2Eq"
        n106 = event-data() -> ()  [unwired: 1 in, 5 out]
        n107 = local write "Inlet LAMBDA"("Inlet LAMBDA") -> ()
        n108 = local write "Inlet O2 (%)"("Inlet O2 (%)") -> ()
        n109 = Decrement(x="Inlet LAMBDA") -> (x-1=w219:T1)
        n110 = Multiply(x=4.76, y="Inlet LAMBDA") -> (x*y=w215:T1)
        n111 = Multiply(x=w219, y=100.0) -> (x*y=w217:T1)
        n112 = Add(x=0.33, y=w215) -> (x+y=w213:T1)
        n113 = Divide(x=w217, y=w213) -> (x/y=w212:T1)
        n114 = Subtract(x="Inlet O2 (%)", y=w212) -> (x-y=w210:T1)
        n115 = Multiply(x=w210, y=2.0) -> (x*y=→"CO Theory (%)":T1)
        n116 = Divide(x=w210, y=4.5) -> (x/y=→"HC Theory (%)":T1)
      }
      event Value Change {
        n117 = event-data() -> ()  [unwired: 1 in, 5 out]
        n118 = local write "NO ppm Loff"("NO ppm Loff") -> ()
        n119 = local write "NO:CO Ratio"("NO:CO Ratio") -> ()
        n120 = Divide(x="NO ppm Loff", y=T1 10000.0) -> (x/y=w222:T1)
        n121 = Multiply(x="NO:CO Ratio", y=w222) -> (x*y=→"CO Theory (%) NO":T1)
      }
      event Value Change {
        n122 = event-data() -> ()  [unwired: 1 in, 5 out]
        n123 = local read "Sample Volume (litres)"() -> (w227:T7)
        n124 = Equal?(x=w227, y=0.0) -> (x = y?=w226:bool)
        n125 = case shown="False" w226 {
          tunnel: w227 -> [w232 _]
          tunnel: "Test Flow Rate(g/s)" -> [w229 _]
          frame False {
            w234 = 60.0 ("y")
            n126 = Multiply(x=w229, y=w234) -> (x*y=w236:T1)
            n127 = Divide(x=w236, y=1.2) -> (x/y=w231:T1)
            "Vol Flow @ STP (l/min)" <- w231
            n128 = Multiply(x=w231, y=w234) -> (x*y=w233:T1)
            n129 = Divide(x=w233, y=w232) -> (x/y=→"Space Velocity (h-1)":T1)
          }
          frame True {
            n130 = One Button Dialog(message="Review sample specification first!") -> ()  [unwired: 1 in, 1 out]
          }
        }
      }
      event "Leak Test": Value Change {
        n131 = event-data() -> ()  [unwired: 1 in, 5 out]
        n132 = flat-sequence {
          tunnel: w239 -> [w242]
          tunnel: [w242] -> w238
          tunnel: w238 -> [w247]
          frame #0 {
            n133 = local write "Test number"(u16 5) -> ()
            n134 = local write "Enum 1"(u16 3 ("Test number")) -> ()
          }
          frame #1 {
            n135 = Enqueue Element(queue=w247, element=Control_3."main" ("Enum")) -> (queue out=w245:refnum<queue>)  [unwired: 2 in, 2 out]
            n136 = Enqueue Element(queue=w245, element=Control_3."start test" ("Enum")) -> (queue out=w244:refnum<queue>)  [unwired: 2 in, 2 out]
            n137 = Enqueue Element(queue=w244, element=Control_3."Leak Test" ("Enum")) -> ()  [unwired: 2 in, 3 out]
          }
        }
      }
      event "Start Test": Value Change {
        n138 = event-data() -> ()  [unwired: 1 in, 6 out]
        n139 = case shown="True" "Start Test" {
          tunnel: w250 -> [_ w259]
          frame False {
          }
          frame True {
            n140 = local read "Log Test Data"() -> (w251:bool)
            n141 = Boolean To (0,1)(Boolean=w251) -> (0, 1=w258:i16)
            n142 = Equal To 0?(x=w258) -> (x = 0?=w257:bool)
            n143 = case shown="True" w257 {
              tunnel: [TRUE ("T button?") w261] -> w252
              frame False {
              }
              frame True {
                # "Log Data Check"
                n144 = Two Button Dialog(message="You are not currently logging data!\nDo you wish to continue?", 1:"No" ("T button name (\"OK\")"), 2:"Yes" ("T button name (\"OK\")")) -> (T button?=w261:bool)
              }
            }
            n145 = Equal?(x=2.0, y=2.0) -> (x = y?=w253:bool)
            n146 = And(x=w253, y=w252) -> (x .and. y?=w254:bool)
            n147 = case shown="True" w254 {
              frame False {
              }
              frame True {
                n148 = flat-sequence {
                  tunnel: "Cycle size" -> [w288]
                  tunnel: [w288] -> w277
                  tunnel: [w291] -> w286
                  tunnel: w277 -> [w291]
                  tunnel: w286 -> [w294]
                  tunnel: [w294] -> w285
                  tunnel: w285 -> [w297]
                  tunnel: [w297] -> w284
                  tunnel: w284 -> [w300]
                  tunnel: [w300] -> w276
                  tunnel: w276 -> [w303]
                  tunnel: [w303] -> w275
                  tunnel: [w306] -> w287
                  tunnel: w275 -> [w306]
                  tunnel: [w309] -> w283
                  tunnel: w287 -> [w309]
                  tunnel: w283 -> [w312]
                  tunnel: [w312] -> w281
                  tunnel: w281 -> [w315]
                  tunnel: [w315] -> w280
                  tunnel: w280 -> [w318]
                  tunnel: [w318] -> w279
                  tunnel: w279 -> [w324]
                  tunnel: [w324] -> w278
                  tunnel: w278 -> [w335]
                  frame #0 {
                    n149 = call-poly <vilib>:"Read From Spreadsheet File.vi"() -> ("all rows"=w289:dbl[][])  [unwired: 7 in, 4 out]
                    n150 = Reshape Array(w289, w288) -> (→"CO":dbl[])
                  }
                  frame #1 {
                    n151 = call-poly <vilib>:"Read From Spreadsheet File.vi"() -> ("all rows"=w293:dbl[][])  [unwired: 7 in, 4 out]
                    n152 = Reshape Array(w293, w291) -> (→"Air Cyc 1":dbl[])
                  }
                  frame #2 {
                    n153 = call-poly <vilib>:"Read From Spreadsheet File.vi"() -> ("all rows"=w295:dbl[][])  [unwired: 7 in, 4 out]
                    n154 = Reshape Array(w295, w294) -> (→"Air Cyc 2":dbl[])
                  }
                  frame #3 {
                    n155 = call-poly <vilib>:"Read From Spreadsheet File.vi"() -> ("all rows"=w299:dbl[][])  [unwired: 7 in, 4 out]
                    n156 = Reshape Array(w299, w297) -> (→"HC Cyc 1":dbl[])
                  }
                  frame #4 {
                    n157 = call-poly <vilib>:"Read From Spreadsheet File.vi"() -> ("all rows"=w302:dbl[][])  [unwired: 7 in, 4 out]
                    n158 = Reshape Array(w302, w300) -> (→"HC Cyc 2":dbl[])
                  }
                  frame #5 {
                    n159 = call-poly <vilib>:"Read From Spreadsheet File.vi"() -> ("all rows"=w304:dbl[][])  [unwired: 7 in, 4 out]
                    n160 = Reshape Array(w304, w303) -> (→"NO":dbl[])
                  }
                  frame #6 {
                    n161 = call-poly <vilib>:"Read From Spreadsheet File.vi"() -> ("all rows"=w307:dbl[][])  [unwired: 7 in, 4 out]
                    n162 = Reshape Array(w307, w306) -> (→"Air Bal":dbl[])
                  }
                  frame #7 {
                    n163 = call-poly <vilib>:"Read From Spreadsheet File.vi"() -> ("all rows"=w311:dbl[][])  [unwired: 7 in, 4 out]
                    n164 = Reshape Array(w311, w309) -> (→"HC Bal":dbl[])
                  }
                  frame #8 {
                    n165 = call-poly <vilib>:"Read From Spreadsheet File.vi"() -> ("all rows"=w313:dbl[][])  [unwired: 7 in, 4 out]
                    n166 = Reshape Array(w313, w312) -> (→"SO Valve 1":dbl[])
                  }
                  frame #9 {
                    n167 = call-poly <vilib>:"Read From Spreadsheet File.vi"() -> ("all rows"=w316:dbl[][])  [unwired: 7 in, 4 out]
                    n168 = Reshape Array(w316, w315) -> (→"SO Valve 2":dbl[])
                  }
                  frame #10 {
                    n169 = call-poly <vilib>:"Read From Spreadsheet File.vi"() -> ("all rows"=w320:dbl[][])  [unwired: 7 in, 4 out]
                    n170 = Reshape Array(w320, w318) -> (→"Open/Closed \nLoop":dbl[])
                  }
                  frame #11 {
                    n171 = local read "Open/Closed \nLoop"() -> (w325:dbl[])
                    n172 = local read "SO Valve 1"() -> (w327:dbl[])
                    n173 = local read "SO Valve 2"() -> (w326:dbl[])
                    n174 = local read "HC Cyc 2"() -> (w330:dbl[])
                    n175 = local read "HC Cyc 1"() -> (w329:dbl[])
                    n176 = local read "Air Cyc 1"() -> (w323:dbl[])
                    n177 = local read "Air Cyc 2"() -> (w328:dbl[])
                    n178 = local read "HC Bal"() -> (w332:dbl[])
                    n179 = local read "Air Bal"() -> (w331:dbl[])
                    n180 = local read "NO"() -> (w321:dbl[])
                    n181 = local read "CO"() -> (w322:dbl[])
                    n182 = Build Array (concatenate)(w324, w322, w323, w328, w329, w330, w321, w331, w332, w327, w326, w325) -> (w333:dbl[])
                    n183 = shared-variable "RT CompactRIO Target 2\\Library 1.lvlib\\Inject_Arrays"(w333) -> ()  [unwired: 1 in, 1 out]
                  }
                  frame #12 {
                    n184 = call-poly <vilib>:"Read From Spreadsheet File.vi"() -> ("all rows"=w336:dbl[][])  [unwired: 7 in, 4 out]
                    n185 = Reshape Array(w336, w335) -> (w334:dbl[])
                    "Lambda" <- w334
                    n186 = shared-variable "RT CompactRIO Target 2\\Library 1.lvlib\\Inject_Arrays_Lambda"(w334) -> ()  [unwired: 1 in, 1 out]
                  }
                }
              }
            }
            n187 = case shown="True" w252 {
              tunnel: w259 -> [_ w266]
              frame False {
              }
              frame True {
                n188 = flat-sequence {
                  tunnel: w266 -> [w269]
                  tunnel: [w269] -> w265
                  tunnel: w265 -> [w273]
                  frame #0 {
                    n189 = local write "Enum 1"(u16 1 ("Test number")) -> ()
                    "Test number" <- "Select Test Type"
                  }
                  frame #1 {
                    n190 = Enqueue Element(queue=w273, element=Control_3."main" ("Enum")) -> (queue out=w271:refnum<queue>)  [unwired: 2 in, 2 out]
                    n191 = property on="Stop Test" class="Bool (strict)"("DisabledEnum"=T11."Enabled" ("Disabled")) -> ()  [unwired: 2 in, 2 out]
                    n192 = Enqueue Element(queue=w271, element=Control_3."start test" ("Enum")) -> ()  [unwired: 2 in, 3 out]
                  }
                }
              }
            }
          }
        }
      }
      event "Log Test Data": Value Change {
        n193 = event-data() -> ()  [unwired: 1 in, 6 out]
        n194 = property on="File Name" class="Str (strict)"() -> ("Value"=w339:T5)  [unwired: 2 in, 2 out]
        n195 = String Length(string=w339) -> (length=w338:i32)
        n196 = Equal To 0?(x=w338) -> (x = 0?=w337:bool)
        n197 = case shown="True" w337 {
          frame False {
          }
          frame True {
            n198 = One Button Dialog(message="A filename has not been entered!") -> ()  [unwired: 1 in, 1 out]
          }
        }
      }
      event "Stop Test": Value Change {
        n199 = event-data() -> ()  [unwired: 1 in, 6 out]
        n200 = case shown="True" "Stop Test" {
          tunnel: w342 -> [_ w344]
          frame False {
          }
          frame True {
            n201 = flat-sequence {
              tunnel: w344 -> [w350]
              tunnel: [w350] -> w348
              tunnel: [w349] -> w347
              tunnel: w348 -> [w354]
              tunnel: [w353] -> w346
              tunnel: w347 -> [w353]
              tunnel: [w352] -> w345
              tunnel: w346 -> [w358]
              tunnel: w345 -> [w357]
              tunnel: [T11."Disabled and Grayed Out" ("Disabled")] -> _
              frame #0 {
                n202 = local read "Connected?"() -> (w349:bool)
                n203 = local write "Stop Cmd"(T1 1.0 ("Stop Cmd")) -> ()
              }
              frame #1 {
                n204 = Enqueue Element(queue=w354, element=Control_3."main" ("Enum")) -> (queue out=w352:refnum<queue>)  [unwired: 2 in, 2 out]
              }
              frame #2 {
                n205 = case shown="True" w358 {
                  tunnel: w357 -> [w359 w362]
                  tunnel: [w359 w361] -> _
                  frame False {
                  }
                  frame True {
                    n206 = local write "Connected?"(FALSE ("Connected?")) -> ()
                    n207 = Enqueue Element(queue=w362, element=Control_3."Multigas disconnect" ("Enum")) -> (queue out=w361:refnum<queue>)  [unwired: 2 in, 2 out]
                  }
                }
              }
            }
            n208 = local write "Start Test"(FALSE ("Start Test")) -> ()
          }
        }
      }
      event "Stopped?": Value Change {
        n209 = event-data() -> ()  [unwired: 1 in, 5 out]
        n210 = flat-sequence {
          tunnel: w366 -> [w370]
          tunnel: [w369] -> w365
          tunnel: [w368] -> w364
          tunnel: w365 -> [w372]
          tunnel: w364 -> [w371]
          frame #0 {
            n211 = local read "Connected?"() -> (w368:bool)
            n212 = Enqueue Element(queue=w370, element=Control_3."main" ("Enum")) -> (queue out=w369:refnum<queue>)  [unwired: 2 in, 2 out]
          }
          frame #1 {
            n213 = case shown="True" w371 {
              tunnel: w372 -> [_ w373]
              frame False {
              }
              frame True {
                n214 = local write "Connected?"(FALSE ("Connected?")) -> ()
                n215 = Enqueue Element(queue=w373, element=Control_3."Multigas disconnect" ("Enum")) -> ()  [unwired: 2 in, 3 out]
              }
            }
          }
        }
      }
      event "Alarm ack": Value Change {
        # "system alarm - set to off"
        n216 = event-data() -> ()  [unwired: 1 in, 5 out]
        n217 = local write "Acknowledge"(TRUE ("Acknowledge")) -> ()
        n218 = property on="Soft Alarm" class="Bool (strict)"("Value"=FALSE ("Acknowledge")) -> ()  [unwired: 2 in, 2 out]
        n219 = property on="Alarm ack" class="Bool"("DisabledEnum"=T11."Disabled and Grayed Out" ("Disabled")) -> ()  [unwired: 2 in, 2 out]
      }
      event "Purge System": Value Change {
        n220 = event-data() -> ()  [unwired: 1 in, 5 out]
        n221 = flat-sequence {
          tunnel: w380 -> [w382]
          tunnel: [w382] -> w379
          tunnel: w379 -> [w383]
          frame #0 {
            n222 = local write "Enum 1"(u16 4 ("Test number")) -> ()
          }
          frame #1 {
            n223 = Enqueue Element(queue=w383, element=Control_3."start test" ("Enum")) -> ()  [unwired: 2 in, 3 out]
          }
        }
      }
      event "Clear log": Value Change {
        n224 = event-data() -> ()  [unwired: 1 in, 5 out]
        n225 = local write "Table"(string[][] [] ("Table")) -> ()
      }
      event "Adv Settings": Value Change {
        # "To be updated"
        # "SO2 conc\nNOx conc\nCO conc\nHC conc\nBleed ratio N2\nBleed ratio CO2"
        n226 = event-data() -> ()  [unwired: 1 in, 6 out]
        n227 = call "Advanced settings MAX.vi"() -> ("output cluster"=→"output cluster":T2)  [unwired: 1 in]
      }
      event "Home": Value Change {
        w388 = FALSE
        n228 = event-data() -> ()  [unwired: 1 in, 6 out]
      }
      event "Performance": Value Change {
        w391 = FALSE
        n229 = event-data() -> ()  [unwired: 1 in, 6 out]
      }
      event "Ageing": Value Change {
        w395 = FALSE
        n230 = event-data() -> ()  [unwired: 1 in, 6 out]
      }
      event "System": Value Change {
        w399 = FALSE
        n231 = event-data() -> ()  [unwired: 1 in, 6 out]
      }
      event "MFC": Value Change {
        w403 = FALSE
        n232 = event-data() -> ()  [unwired: 1 in, 6 out]
      }
      event "Analyser": Value Change {
        w408 = FALSE
        n233 = event-data() -> ()  [unwired: 1 in, 6 out]
      }
      event "Alarm": Value Change {
        w411 = FALSE
        n234 = event-data() -> ()  [unwired: 1 in, 6 out]
      }
    }
    "stop 2" <- w69
    n235 = local write "Tab Control"(w67) -> ()
    n236 = case shown="False" w66 {
      tunnel: [w81 w89] -> w68
      tunnel: w67 -> [w81 _]
      tunnel: w65 -> [_ w89]
      tunnel: w64 -> [_ w88]
      tunnel: w63 -> [_ w87]
      tunnel: w62 -> [_ w86]
      tunnel: w61 -> [_ w85]
      tunnel: w60 -> [_ w84]
      tunnel: w59 -> [_ w83]
      tunnel: w58 -> [_ w82]
      tunnel: [w79 w88] -> w57
      tunnel: [w78 w87] -> w56
      tunnel: [w74 w86] -> w55
      tunnel: [w75 w85] -> w54
      tunnel: [w76 w84] -> w53
      tunnel: [w77 w83] -> w52
      tunnel: [w80 w82] -> w51
      tunnel: w50 -> [w79 _]
      tunnel: w49 -> [w78 _]
      tunnel: w48 -> [w80 _]
      tunnel: w47 -> [w77 _]
      tunnel: w46 -> [w76 _]
      tunnel: w45 -> [w75 _]
      tunnel: w44 -> [w74 _]
      frame False {
      }
      frame True {
      }
    }
    n237 = local write "Home"(w57) -> ()
    n238 = local write "Performance"(w56) -> ()
    n239 = local write "Ageing"(w55) -> ()
    n240 = local write "System"(w54) -> ()
    n241 = local write "MFC"(w53) -> ()
    n242 = local write "Analyser"(w52) -> ()
    n243 = local write "Alarm"(w51) -> ()
  }
  n244 = node-c288(nitl_modes."Discard missed periods, maintain original phase" ("Mode")) -> (w15:T12)  [unwired: 4 in]
  n245 = node-c288(i64 100 ("Period")) -> (w8:T12)  [unwired: 3 in]
  n246 = timed-loop {
    timing: w15 -> [_]
    timing-out: [_] -> w14
    shift-right: [w548] -> _
    shift-left: path "" -> [w515]
    shift-right: [w606] -> _
    shift-left: w9 -> [w640]
    shift-right: [w416] -> _
    shift-left: _ -> [w616]
    shift-right: [w596] -> _
    shift-left: w9 -> [w599]
    shift-right: [w597] -> _
    shift-left: w9 -> [w598]
    shift-right: [w540] -> _
    shift-left: 0 ("t") -> [w539]
    shift-right: [w530] -> _
    shift-left: _ -> [w519]
    shift-right: [w529] -> _
    shift-left: _ -> [w520]
    shift-right: [w528] -> _
    shift-left: _ -> [w521]
    shift-right: [w527] -> _
    shift-left: _ -> [w522]
    shift-right: [w526] -> _
    shift-left: _ -> [w523]
    shift-right: [w525] -> _
    shift-left: _ -> [w524]
    shift-right: [w505] -> _
    shift-left: _ -> [w506]
    stop <- w639 stop-if-true
    w555 = 54321.0 ("y")
    # "56 first gas"
    # "Flow Rate Guide"
    # "Temperature Guide"
    # "0   Flow Rate 1\n1   Flow Rate 2\n     ECM 1\n     ECM 2\n2   CO2 U\n3   CO U\n4   HC U\n5   O2 U\n7   CO2 D\n8   CO D\n9   HC D\n10 O2 D\n12 TC1X\n13 TC2A\n14 TC3Y\n15 TC4B\n16 TC5\n17 TC6\n32 Venturi 1\n33 Venturi 2\n34 Tank\n35 Bearing 1\n36 Bearing 2\n38 Ex A\n39 Ex B\n40 Ex C\n41 Ex D\n     MFC Box\n42 Furnace 1\n43 Furnace 2\n44 NO 1 ?? \n45 Lambda 1\n46 NO 2 ??\n47 Lambda 2\n56 CO (L)\n57 CO (H)\n58CO2\n59 O2\n60 THC\n61 NO\n62 NOx\n63 NO2"
    n247 = node-c288() -> (→"Finished Late? [i-1]":bool, →"Iteration Duration":i64)  [unwired: 1 in, 1 out]
    n248 = shared-variable "RT CompactRIO Target 2\\Library 1.lvlib\\DATA"() -> (w638:dbl[])  [unwired: 1 in, 1 out]
    n249 = local read "MKS"() -> (w436:bool)
    n250 = Type Cast(type=w638, x=w638) -> (*(type *) &x=w648:dbl[])
    n251 = local read "Advanced Logging"() -> (w552:bool)
    n252 = Delete From Array(array=w648, length=4, index=0) -> (deleted portion=w645:dbl[], array with subset deleted=w431:dbl[])
    n253 = call "MKS.vi"("IP Address"="192.168.1.5", "Connect"=w436) -> ("Emissions"=w517:dbl[])  [unwired: 9 in]
    n254 = call "MKS.vi"("IP Address"="192.168.254.2", "Connect"=FALSE) -> ("Emissions"=w518:dbl[])  [unwired: 9 in]
    n255 = local read "Full System"() -> (w547:bool)
    n256 = Index Array(array=w517, index=0) -> (element=w559:dbl)
    n257 = Index Array(array=w518, index=0) -> (element=w557:dbl)
    n258 = case shown="True" w552 {
      tunnel: [w746 w797] -> w553
      tunnel: w431 -> [w747 w797]
      tunnel: [w745 "Time\tFlow 1 g/s\tFlow 2 g/sLambda 1\tLambda 2\tLambda 3\tLambda 4\tTank P\tTC1X\tTC2A\tTCY\tTC4B\tTC5\tTC6\tTC7\tTC8\tTC9\tTC10\tTC11\tTC12\tTC13\tMFC Box\tMFC Box 2\tCabinet Temp\tTC17\tTC18\tTC19\tTC20\tTC Vent 1\tTC Vent 2\tTC Tank\tTC Fan B1\tTC Fan B2\tTC Cab\tTC Ex A\tTC Ex B\tTC Ex C\tTC Ex D\tSpare\tTC Furn 1\tTC Furn 2\tRapidox\tCO2\tCO\tTHC\tO2\t\tNOx\tCO2\tCO\tTHC\tNOx\tEmisions Switch 1\tFur Lambda 1\tFur Lambda 2\tNOx 1\tO2 1\tLambda N1\tNOx 2\tO2 2\tLambda N2\tLeak Test\tHeat Load 1\tHeatLoad 2\tHeat Load 3\tHeat Load 4\tCOH\tCO2\tCOL\tO2\tSO2\tTHC\tNOx\r\n" ("Heading string 2")] -> w551
      tunnel: w547 -> [w744 _]
      frame False {
        n259 = case shown="True" w744 {
          tunnel: w747 -> [w762 w777]
          tunnel: [w753 w779] -> w746
          tunnel: ["Time\tFlow 1 g/s\tCO2 U %\tCO U %\tHC U ppm\tO2 U %\tNO U ppm\tCO2 D %\tCO D %\tHC D ppm\tO2 D %\tNO D ppm\tTC1X\tTC2A\tTCY\tTC4B\tTC5\tTC6\tTC7\tTC8\tRapidox\tLambda 1\tLambda 2\tNOX 1 ppm\tNOX 2 ppm\tUEGO 1\tUEGO 2" ("Heading string 2") "Time\tFlow 1 g/s\tFlow 2 g/s\tCO2 U %\tCO U %\tHC U ppm\tO2 U %\tNO U ppm\tCO2 D %\tCO D %\tHC D ppm\tO2 D %\tNO D ppm\tTC1X\tTC2A\tTCY\tTC4B\tTC5\tTC6\tTC7\tTC8\tRapidox\tLambda 1\tLambda 2\tNOX 1 ppm\tNOX 2 ppm\tUEGO 1\tUEGO 2" ("Heading string 2")] -> w745
          frame False {
            n260 = Delete From Array(array=w762, length=21, index=0) -> (deleted portion=w749:dbl[], array with subset deleted=w761:dbl[])
            n261 = Index Array(array=w761, index #1=47 ("index"), index #2=48 ("index"), index #3=49 ("index"), index #4=50 ("index"), index #5=51 ("index"), index #6=52 ("index"), index #7=53 ("index")) -> (element #1=w760:dbl, element #2=w759:dbl, element #3=w758:dbl, element #4=w757:dbl, element #5=w756:dbl, element #6=w755:dbl, element #7=w754:dbl)
            n262 = Delete From Array(array=w749, length=1, index=2) -> (array with subset deleted=w748:dbl[])  [unwired: 1 out]
            n263 = Build Array (concatenate)(w748, w760, w759, w758, w757, w756, w755, w754) -> (w753:dbl[])
          }
          frame True {
            n264 = Delete From Array(array=w777, length=21, index=0) -> (deleted portion=w774:dbl[], array with subset deleted=w778:dbl[])
            n265 = Index Array(array=w778, index #1=47 ("index"), index #2=48 ("index"), index #3=49 ("index"), index #4=50 ("index"), index #5=51 ("index"), index #6=52 ("index"), index #7=53 ("index")) -> (element #1=w786:dbl, element #2=w785:dbl, element #3=w784:dbl, element #4=w783:dbl, element #5=w782:dbl, element #6=w781:dbl, element #7=w780:dbl)
            n266 = Delete From Array(array=w774, length=2, index=1) -> (array with subset deleted=w772:dbl[])  [unwired: 1 out]
            n267 = Build Array (concatenate)(w772, w786, w785, w784, w783, w782, w781, w780) -> (w779:dbl[])
          }
        }
      }
      frame True {
      }
    }
    n268 = Not Equal?(x=w559, y=w555) -> (x != y?=w558:bool)
    n269 = Not Equal?(x=w555, y=w557) -> (x != y?=w556:bool)
    n270 = Index Array(array=w645) -> (element #1=w416:dbl, element #2=w619:dbl, element #3=w434:dbl, element #4=w615:dbl)  [unwired: 4 in]
    "Error" <- w434
    n271 = Equal?(x=w416, y=4.0) -> (x = y?=w418:bool)
    n272 = Equal?(x=w416, y=5.0) -> (x = y?=w417:bool)
    n273 = Or(x=w418, y=w417) -> (x .or. y?=w415:bool)
    n274 = case shown="True" w415 {
      frame False {
      }
      frame True {
        n275 = local write "Start Test"(FALSE ("Start Test")) -> ()
        n276 = local write "Enum 1"(i16 0 ("Enum 1")) -> ()
      }
    }
    n277 = case shown="False" w558 {
      tunnel: [w803 w814] -> w516
      tunnel: w518 -> [w802 w813]
      tunnel: w517 -> [_ w812]
      tunnel: w556 -> [w801 w811]
      tunnel: [w800 w808] -> w554
      frame False {
        n278 = case shown="False" w801 {
          tunnel: [dbl[] [54321.0] w807] -> w803
          tunnel: w802 -> [_ w807]
          tunnel: ["\r\n" ("Heading string 2") "\tNO\tNO2 (150)\tNO2 (2000)\tN2O\tNH3 (300)\tNH3 (3000)\tHNCO (400)\tH2O\tCO2\tCO (500)\tCO (1)\tCH4 (250)\tCH4 (3000)\tNOxP\tPropane\r\n" ("Heading string 2")] -> w798
          frame False {
          }
          frame True {
          }
        }
        n279 = Build Array(" " ("Heading string 2"), w798) -> (w800:string[])
      }
      frame True {
        n280 = case shown="True" w811 {
          tunnel: [w816 w820] -> w814
          tunnel: w813 -> [_ w819]
          tunnel: w812 -> [w816 w818]
          tunnel: ["\rn" ("Heading string 2") "\tNO\tNO2 (150)\tNO2 (2000)\tN2O\tNH3 (300)\tNH3 (3000)\tHNCO (400)\tH2O\tCO2\tCO (500)\tCO (1)\tCH4 (250)\tCH4 (3000)\tNOxP\tPropane\r" ("Heading string 2")] -> w809
          frame False {
          }
          frame True {
            n281 = Build Array (concatenate)(w818, w819) -> (w820:dbl[])
          }
        }
        n282 = Build Array("\tNO\tNO2 (150)\tNO2 (2000)\tN2O\tNH3 (300)\tNH3 (3000)\tHNCO (400)\tH2O\tCO2\tCO (500)\tCO (1)\tCH4 (250)\tCH4 (3000)\tNOxP\tPropane" ("Heading string 2"), w809) -> (w808:string[])
      }
    }
    n283 = To Unsigned Long Integer(number=w615) -> (unsigned 32bit integer=w614:u32)
    n284 = Number To Boolean Array(number=w614) -> (Boolean array=w628:bool[])
    n285 = Index Array(array=w628) -> (element #2=w626:bool, element #3=w625:bool, element #4=w611:bool, element #5=→"ExtAnUp":bool, element #6=→"ExtAnDn":bool)  [unwired: 6 in, 1 out]
    "Extractor Fan On" <- w611
    n286 = case shown="0, Default" w619 {
      tunnel: [w840 TRUE FALSE] -> w618
      tunnel: [w841 FALSE TRUE] -> w617
      frame 0, Default {
        n287 = local read "Pass"() -> (w841:bool)
        n288 = local read "Fail"() -> (w840:bool)
      }
      frame 1 {
      }
      frame 2 {
      }
    }
    "Pass" <- w617
    "Fail" <- w618
    n289 = Or(x=w626, y=w625) -> (x .or. y?=→"Doors Open":bool)
    n290 = Not(x=w611) -> (.not. x?=→"Doors Unlocked":bool)
    n291 = Less?(x=w416, y=w616) -> (x < y?=w613:bool)
    n292 = Path To String(path="File Path") -> (string=w609:string)
    n293 = local read "Connected"() -> (w612:bool)
    n294 = Concatenate Strings(w609, "\\" ("string"), "File Name") -> (w562:string)
    n295 = call "Mexa_7170.vi"("String 1 In"=w523, "Connect"=FALSE, "connection ID 1 In"=w522, "error out 1 In"=w521, "connection ID 2 In"=w520, "error out 2 In"=w519, "Time In"=w524) -> ("Emissions"=→"Emissions":dbl[], "String 1 Out"=w526:string, "connection ID 1 Out"=w527:refnum<k5>, "error 1 out"=w528:errorcluster, "connection ID 2 Out"=w529:refnum<k16>, "Time Out"=w525:i16, "error 2 out"=w530:errorcluster)  [unwired: 2 in]
    n296 = And(x=w612, y=w613) -> (x .and. y?=w605:bool)
    n297 = local read "Mexa_One Emissions"() -> (w422:dbl[])
    n298 = Build Array (concatenate)(w422, w516) -> (w429:dbl[])
    n299 = local write "Stopped?"(w605) -> ()
    n300 = Build Array (concatenate)(w431, w429) -> (w430:dbl[])
    n301 = Equal To 0?(x=w434) -> (x = 0?=w550:bool)
    n302 = Equal To 0?(x=w416) -> (x = 0?=w549:bool)
    n303 = Build Array (concatenate)(w553, w429) -> (w641:dbl[])
    n304 = Equal?(x=w416, y=2.0) -> (x = y?=w570:bool)
    n305 = String To Path(string=w562) -> (path=w607:path)
    n306 = Build Array(w550, w549) -> (w623:bool[])
    n307 = Equal?(x=w416, y=3.0) -> (x = y?=w567:bool)
    n308 = Equal?(x=w416, y=4.0) -> (x = y?=w565:bool)
    n309 = Boolean Array To Number(Boolean array=w623) -> (number=w622:u32)
    n310 = Index Array(array=w430, index=6) -> (element=→"Pressure":dbl)
    n311 = Not Equal?(x=w607, y=w515) -> (x != y?=w650:bool)
    n312 = Compound Arithmetic op=OR(w570, w567, w565) -> (w569:bool)
    n313 = case shown="3" w622 {
      tunnel: [w866 w867 w872 w874] -> _
      tunnel: [w866 w867 w872 w874] -> _
      tunnel: [w866 w867 w872 w874] -> w621
      tunnel: [w866 w867 w870 w874] -> w620
      tunnel: [T11."Enabled" ("Disabled") T11."Enabled" ("Disabled") w870 w874] -> _
      tunnel: [FALSE FALSE FALSE TRUE] -> w604
      frame 0, Default {
        w866 = T11."Disabled and Grayed Out" ("Disabled")
      }
      frame 1 {
        w867 = T11."Disabled and Grayed Out" ("Disabled")
      }
      frame 2 {
        w870 = T11."Enabled" ("Disabled")
        w872 = T11."Disabled and Grayed Out" ("Disabled")
      }
      frame 3 {
        w874 = T11."Enabled" ("Disabled")
        (unwired) T11."Disabled and Grayed Out" ("Disabled")
      }
    }
    n314 = local read "Log Test Data"() -> (w563:bool)
    n315 = for {
      tunnel: w641 -> [w882] mode=indexing
      tunnel: [w881] -> w652 mode=indexing
      n316 = Number To Fractional String(number=w882, precision (6)=i16 3) -> (F-format string=w881:string)  [unwired: 2 in]
    }
    n317 = Select(t=w607, s=w650, f=w515) -> (s? t:f=w651:path)
    n318 = And(x=w563, y=w569) -> (x .and. y?=w666:bool)
    "Log?" <- w666
    n319 = case shown="True" w650 {
      tunnel: w651 -> [w875 w880]
      tunnel: [w875 w879] -> w649
      tunnel: w554 -> [_ w877]
      tunnel: w551 -> [_ w876]
      frame False {
      }
      frame True {
        # "setting up the header"
        n320 = Build Array (concatenate)(w876, w877) -> (w878:string[])
        n321 = call-poly <vilib>:"Write To Spreadsheet File.vi"("1D data"=w878, "file path (dialog if empty)"=w880) -> ("new file path (Not A Path if cancelled)"=w879:path)  [unwired: 6 in]
      }
    }
    n322 = Equal?(x=w416, y=0.0) -> (x = y?=w593:bool)
    n323 = case shown="0, Default" w416 {
      tunnel: [w827 w829 w832 w833 TRUE FALSE] -> w445
      tunnel: [w827 w829 w832 TRUE w835 w838] -> w443
      tunnel: [TRUE w829 w832 w833 w835 w838] -> w442
      tunnel: [w827 TRUE TRUE w833 w835 w838] -> w426
      frame 0, Default {
        w827 = FALSE
      }
      frame 1 {
        w829 = FALSE
      }
      frame 2 {
        w832 = FALSE
      }
      frame 3 {
        w833 = FALSE
      }
      frame 4 {
        w835 = FALSE
        n324 = local write "Stop Cmd"(T1 0.0 ("Stop Cmd")) -> ()
      }
      frame 5 {
        w838 = FALSE
      }
    }
    n325 = property class="VI"("Front Panel.Closeable"=w604) -> ()  [unwired: 2 in, 2 out]
    n326 = property on="Compile Test Button" class="Bool"("DisabledEnum"=w621) -> ()  [unwired: 2 in, 2 out]
    n327 = property on="Purge System" class="Bool"("DisabledEnum"=w620) -> ()  [unwired: 2 in, 2 out]
    n328 = local read "Full System"() -> (w594:bool)
    n329 = Index Array(array=w429, index #1=0 ("index"), index #2=1 ("index"), index #3=2 ("index"), index #4=3 ("index")) -> ()  [unwired: 4 out]
    n330 = Equal?(x=w434, y=1024.0) -> (x = y?=w432:bool)
    n331 = case shown="False" "Demo On" {
      tunnel: w445 -> [w672 w676]
      tunnel: [w672 w675] -> w444
      tunnel: w443 -> [w674 _]
      tunnel: w442 -> [w673 _]
      tunnel: [w673 w675] -> w441
      tunnel: [w674 TRUE] -> w440
      tunnel: [w672 w676] -> w428
      tunnel: [w671 w675] -> w427
      tunnel: w426 -> [w671 _]
      frame False {
      }
      frame True {
        w675 = FALSE
      }
    }
    "Cool Down" <- w444
    "Test In Progress" <- w440
    "Standby" <- w441
    "Warm Up" <- w427
    n332 = case shown="False" w432 {
      tunnel: w434 -> [w669 _]
      tunnel: [w669 0.0 ("Numeric")] -> w435
      frame False {
      }
      frame True {
      }
    }
    n333 = Build Array(w594, w593) -> (w595:bool[])
    n334 = local write "Stop Test"(w428) -> ()
    n335 = Boolean Array To Number(Boolean array=w595) -> (number=w592:u32)
    n336 = call "Demo_Guide.vi"("Time In"=w506, "Temperature Sync"="Demo Sync", "Duration -1"="Duration -1", "TempGuide"="Demo On") -> ("Output array"=w481:dbl[], "Time out"=w505:i32)  [unwired: 6 in]
    n337 = Not Equal To 0?(x=w435) -> (x != 0?=w643:bool)
    n338 = Not Equal?(x=w435, y=w640) -> (x != y?=w642:bool)
    n339 = case shown="False" w666 {
      tunnel: w649 -> [w886 w894]
      tunnel: [w886 w906] -> w548
      tunnel: w652 -> [_ w902]
      tunnel: w599 -> [_ w895]
      tunnel: w598 -> [w885 w890]
      tunnel: [w885 w892] -> w597
      tunnel: [w884 w891] -> w596
      frame False {
        n340 = local read "Log interval (seconds)"() -> (w884:T1)
      }
      frame True {
        n341 = Get Date/Time In Seconds() -> (seconds since 1Jan1904=w903:timestamp)
        n342 = Decrement(x=w895) -> (x-1=w896:T1)
        n343 = Less Than 0?(x=w896) -> (x < 0?=w897:bool)
        n344 = Equal To 0?(x=w896) -> (x = 0?=w898:bool)
        n345 = Build Array(w897, w898) -> (w899:bool[])
        n346 = Path To String(path=w894) -> (string=w889:string)
        "File name" <- w889
        n347 = Format Date/Time String(time format string (%c)="%d/%m/%y %H:%M:%S", seconds (now)=w903) -> (date/time string=w904:string)  [unwired: 1 in]
        n348 = Boolean Array To Number(Boolean array=w899) -> (number=w900:u32)
        n349 = case shown="2" w900 {
          tunnel: w895 -> [w913 w914 _]
          tunnel: [w912 w914 w917] -> w891
          tunnel: w889 -> [w911 w916 w920]
          tunnel: [w908 w916 w918] -> w893
          tunnel: [w907 w915 w919] -> w892
          tunnel: w890 -> [w907 w915 w923]
          frame 0, Default {
            n350 = Number To Decimal String(number=w907) -> (decimal integer string=w909:string)  [unwired: 1 in]
            n351 = call <vilib>:"Space Constant.vi"() -> ("String"=w910:string)
            n352 = Decrement(x=w913) -> (x-1=w912:T1)
            n353 = Concatenate Strings(w911, w910, w909) -> (w908:string)
          }
          frame 1 {
          }
          frame 2 {
            n354 = Increment(x=w923) -> (x+1=w919:dbl)
            n355 = local read "Log interval (seconds)"() -> (w917:T1)
            n356 = Number To Decimal String(number=w919) -> (decimal integer string=w921:string)  [unwired: 1 in]
            n357 = call <vilib>:"Space Constant.vi"() -> ("String"=w922:string)
            n358 = Concatenate Strings(w920, w922, w921) -> (w918:string)
          }
        }
        n359 = Build Array (concatenate)(w904, w902) -> (w888:string[])
        n360 = String To Path(string=w893) -> (path=w887:path)
        n361 = call-poly <vilib>:"Write To Spreadsheet File.vi"("append to file? (new file:F)"=TRUE, "1D data"=w888, "file path (dialog if empty)"=w887) -> ("new file path (Not A Path if cancelled)"=w906:path)  [unwired: 5 in]
      }
    }
    n362 = And(x=w643, y=w642) -> (x .and. y?=w644:bool)
    n363 = Index Array(array=w430, index #1=0 ("index"), index #2=1 ("index"), index #3=68 ("index"), index #4=65 ("index"), index #5=42 ("index"), index #6=44 ("index"), index #7=45 ("index"), index #8=47 ("index"), index #9=70 ("index"), index #10=46 ("index"), index #11=7 ("index"), index #12=8 ("index"), index #13=9 ("index"), index #14=10 ("index"), index #15=11 ("index"), index #16=12 ("index"), index #17=27 ("index"), index #18=28 ("index"), index #19=29 ("index"), index #20=30 ("index"), index #21=31 ("index"), index #22=32 ("index"), index #23=33 ("index"), index #24=34 ("index"), index #25=35 ("index"), index #26=38 ("index"), index #27=39 ("index"), index #28=70 ("index"), index #29=100 ("index"), index #30=2 ("index"), index #31=3 ("index"), index #32=4 ("index"), index #33=5 ("index")) -> (element #1=w542:dbl, element #2=w541:dbl, element #3=w504:dbl, element #4=w502:dbl, element #5=w500:dbl, element #6=w499:dbl, element #7=w498:dbl, element #8=w497:dbl, element #9=w496:dbl, element #10=w494:dbl, element #11=w493:dbl, element #12=w491:dbl, element #13=w489:dbl, element #14=w487:dbl, element #15=w485:dbl, element #16=w483:dbl, element #17=w476:dbl, element #18=w474:dbl, element #19=w472:dbl, element #20=w470:dbl, element #21=w468:dbl, element #22=w466:dbl, element #23=w464:dbl, element #24=w462:dbl, element #25=w460:dbl, element #26=→"Furnace temp 1":dbl, element #27=→"Furnace temp 2":dbl, element #28=w458:dbl, element #29=w456:dbl, element #30=w454:dbl, element #31=w452:dbl, element #32=w450:dbl, element #33=w448:dbl)
    n364 = case shown="False" w644 {
      tunnel: w435 -> [w847 w859]
      tunnel: w642 -> [w850 _]
      tunnel: [w846 w859] -> w606
      frame False {
        n365 = Equal To 0?(x=w847) -> (x = 0?=w851:bool)
        n366 = And(x=w851, y=w850) -> (x .and. y?=w849:bool)
        n367 = case shown="True" w849 {
          frame False {
          }
          frame True {
            w854 = FALSE ("Ack hard alarm!")
            n368 = property on="Hard Alarm" class="Bool (strict)"("Value"=w854) -> ()  [unwired: 2 in, 2 out]
            n369 = property on="System Alarm" class="Bool (strict)"("Value"=w854) -> ()  [unwired: 2 in, 2 out]
            n370 = property on="System Alarm" class="Bool (strict)"("Value"=w854) -> ()  [unwired: 2 in, 2 out]
          }
        }
        n371 = case shown="True" "Acknowledge" {
          tunnel: [w852 0.0 ("Numeric")] -> w846
          tunnel: w847 -> [w852 _]
          frame False {
          }
          frame True {
          }
        }
      }
      frame True {
        n372 = local read "Table"() -> (w862:string[][])
        n373 = call "Error list.vi"("Error code"=w859, "Error array in"=w862) -> ("Hard alarm?"=w856:bool, "Error array out"=w861:string[][])  [unwired: 8 in]
        "Hard Alarm" <- w856
        n374 = Not(x=w856) -> (.not. x?=w857:bool)
        "Soft Alarm" <- w857
        n375 = Or(x=w857, y=w856) -> (x .or. y?=→"System Alarm":bool)
        n376 = case shown="True" w857 {
          frame False {
          }
          frame True {
            n377 = property on="Alarm ack" class="Bool"("DisabledEnum"=T11."Enabled" ("Disabled")) -> ()  [unwired: 2 in, 2 out]
          }
        }
        n378 = local write "Table"(w861) -> ()
        n379 = local write "Acknowledge"(FALSE ("Acknowledge")) -> ()
        n380 = property on="Tab Control" class="TabCtl (strict)"("Value"=6) -> ()  [unwired: 2 in, 2 out]
      }
    }
    n381 = case shown="1" w592 {
      tunnel: w542 -> [w822 w824 _ _]
      tunnel: w541 -> [_ w823 _ _]
      tunnel: [w822 w824 w825 w826] -> w480
      tunnel: [0.0 ("y") w823 w825 w826] -> w478
      frame 0, Default {
      }
      frame 1 {
      }
      frame 2 {
        w825 = 0.0 ("y")
      }
      frame 3 {
        w826 = 0.0 ("y")
      }
    }
    n382 = case shown="False" "Demo On" {
      tunnel: w504 -> [w708 _]
      tunnel: [w708 w740] -> w503
      tunnel: w502 -> [w707 _]
      tunnel: [w707 w710] -> w501
      tunnel: w500 -> [w706 _]
      tunnel: [w706 w717] -> _
      tunnel: w499 -> [w705 _]
      tunnel: [w705 w717] -> _
      tunnel: w498 -> [w704 _]
      tunnel: [w704 w717] -> _
      tunnel: w497 -> [w703 _]
      tunnel: [w703 w717] -> _
      tunnel: [w702 w738] -> w495
      tunnel: w496 -> [w702 _]
      tunnel: w494 -> [w701 _]
      tunnel: [w701 w717] -> _
      tunnel: w493 -> [w700 _]
      tunnel: [w700 w736] -> w492
      tunnel: w491 -> [w699 _]
      tunnel: [w699 w734] -> w490
      tunnel: w489 -> [w698 _]
      tunnel: [w698 w717] -> w488
      tunnel: w487 -> [w697 _]
      tunnel: [w697 w717] -> w486
      tunnel: w485 -> [w696 _]
      tunnel: [w696 w717] -> w484
      tunnel: w483 -> [w695 _]
      tunnel: [w695 w717] -> w482
      tunnel: w481 -> [_ w743]
      tunnel: w480 -> [w694 _]
      tunnel: [w694 w742] -> w479
      tunnel: w478 -> [w693 _]
      tunnel: [w693 w717] -> w477
      tunnel: w476 -> [w692 _]
      tunnel: [w692 w732] -> w475
      tunnel: w474 -> [w691 _]
      tunnel: [w691 w717] -> w473
      tunnel: w472 -> [w690 _]
      tunnel: [w690 w730] -> w471
      tunnel: w470 -> [w689 _]
      tunnel: [w689 w728] -> w469
      tunnel: w468 -> [w688 _]
      tunnel: [w688 w726] -> w467
      tunnel: w466 -> [w687 _]
      tunnel: [w687 w724] -> w465
      tunnel: w464 -> [w686 _]
      tunnel: [w686 w722] -> w463
      tunnel: w462 -> [w685 _]
      tunnel: [w685 w720] -> w461
      tunnel: w460 -> [w684 _]
      tunnel: [w684 w719] -> w459
      tunnel: w458 -> [w683 _]
      tunnel: [w683 w718] -> w457
      tunnel: w456 -> [w682 _]
      tunnel: [w682 w717] -> w455
      tunnel: w454 -> [w681 _]
      tunnel: [w681 w715] -> w453
      tunnel: w452 -> [w680 _]
      tunnel: [w680 w716] -> w451
      tunnel: w450 -> [w679 _]
      tunnel: [w679 w716] -> w449
      tunnel: w448 -> [w678 _]
      tunnel: [w678 w716] -> w447
      frame False {
      }
      frame True {
        w716 = 5.0 ("Numeric")
        w717 = 0.0 ("Numeric")
        n383 = Index Array(array=w743, index #1=2 ("index"), index #2=13 ("index"), index #3=14 ("index"), index #4=0 ("index"), index #5=1 ("index"), index #6=4 ("index"), index #7=5 ("index"), index #8=6 ("index"), index #9=7 ("index"), index #10=8 ("index"), index #11=9 ("index"), index #12=10 ("index"), index #13=11 ("index"), index #14=15 ("index"), index #15=3 ("index"), index #16=12 ("index")) -> (element #1=w742:dbl, element #2=w740:dbl, element #3=w738:dbl, element #4=w736:dbl, element #5=w734:dbl, element #6=w732:dbl, element #7=w730:dbl, element #8=w728:dbl, element #9=w726:dbl, element #10=w724:dbl, element #11=w722:dbl, element #12=w720:dbl, element #13=w719:dbl, element #14=w718:dbl, element #15=w715:dbl, element #16=w710:dbl)
      }
    }
    n384 = call "Flow_Guide-plot.vi"("Temperature Sync"="Flow Sync", "Temp Band % (e.g. 1%=1.01)"="Flow Band %", "Mean(Off)/Interval(On)"="Mean(Off)/Interval(On) 2", "Guide"="FlowGuide") -> ()  [unwired: 5 in, 3 out]
    n385 = Merge Signals(w495) -> (→"HC Concentration (ppm)":dynamicdata)
    n386 = Merge Signals(w475, w473, w471, w469, w467) -> (→"System Temperatures (°C)":dynamicdata)
    n387 = Merge Signals(w465, w463, w461, w459) -> (→"Heat Exchanger Temperatures (°C)":dynamicdata)
    n388 = Merge Signals(w457, w455) -> (→"NO Concentration (ppm)":dynamicdata)
    n389 = Merge Signals(w453, w451, w449, w447) -> (→"Lambda":dynamicdata)
    n390 = Merge Signals(w479, w477) -> (→"Flow Rate (g/s)":dynamicdata)
    n391 = Merge Signals(w503, w501) -> (→"O2/CO Concentration":dynamicdata)
    n392 = call "Temp_Guide-plot.vi"("Time In"=w539, "Temperature Sync"="Temperature Sync", "Temp Band % (e.g. 1%=1.01)"="Temp Band %", "Mean(Off)/Interval(On)"="Mean(Off)/Interval(On)", "TempGuide"="TempGuide") -> ("Graph 4"=w538:dbl, "Graph 3"=w537:dbl, "Graph 2"=w536:dbl, "Graph 1"=w535:dbl, "Time out"=w540:i32)  [unwired: 2 in]
    n393 = local read "stop 2"() -> (w639:bool)
    n394 = Merge Signals(w492, w490, w488, w486, w484, w482, w535, w536, w537, w538) -> (→"Sample Temperatures (°C)":dynamicdata)
    n395 = node-c288() -> ()  [unwired: 1 in, 1 out]
  }
  n396 = timed-loop {
    timing: w8 -> [_]
    timing-out: [_] -> w7
    shift-right: [w941] -> _
    shift-left: _ -> [w940]
    shift-right: [w939] -> _
    shift-left: _ -> [w938]
    shift-right: [w936] -> _
    shift-left: _ -> [w937]
    shift-right: [w934] -> _
    shift-left: _ -> [w929]
    shift-right: [w935] -> _
    shift-left: _ -> [w930]
    shift-right: [w933] -> _
    shift-left: _ -> [w931]
    stop <- _ stop-if-true
    n397 = node-c288() -> ()  [unwired: 1 in, 1 out]
    n398 = shared-variable "RT CompactRIO Target 2\\Library 1.lvlib\\DATA_2"() -> (w959:dbl[])  [unwired: 1 in, 1 out]
    n399 = call "Mexa_One.vi"() -> ()  [unwired: 9 in, 7 out]
    n400 = local read "Mexa One"() -> (w932:bool)
    n401 = case shown="\"CO\", Default" "Graph 1 Box" {
      tunnel: [0 ("index") 1 ("index") 2 ("index") 3 ("index") 4 ("index") 5 ("index") 6 ("index") 7 ("index")] -> w960
      tunnel: [8 ("index") 9 ("index") 10 ("index") 11 ("index") 12 ("index") 13 ("index") 14 ("index") 15 ("index")] -> w967
      frame "CO", Default {
      }
      frame "HC Cycle 1" {
      }
      frame "Air Cycle 1" {
      }
      frame "NO" {
      }
      frame "Air Bal" {
      }
      frame "HC Bal" {
      }
      frame "Air Cycle 2" {
      }
      frame "HC Cycle 2" {
      }
    }
    n402 = case shown="\"Air Cycle 2\"" "Graph 2 Box" {
      tunnel: [0 ("index") 1 ("index") 2 ("index") 3 ("index") 4 ("index") 5 ("index") 6 ("index") 7 ("index")] -> w951
      tunnel: [8 ("index") 9 ("index") 10 ("index") 11 ("index") 12 ("index") 13 ("index") 14 ("index") 15 ("index")] -> w952
      frame "CO" {
      }
      frame "HC Cycle 1", Default {
      }
      frame "Air Cycle 1" {
      }
      frame "NO" {
      }
      frame "Air Bal" {
      }
      frame "HC Bal" {
      }
      frame "Air Cycle 2" {
      }
      frame "HC Cycle 2" {
      }
    }
    n403 = case shown="\"Air Cycle 1\", Default" "Graph 3 Box" {
      tunnel: [0 ("index") 1 ("index") 2 ("index") 3 ("index") 4 ("index") 5 ("index") 6 ("index") 7 ("index")] -> w949
      tunnel: [8 ("index") 9 ("index") 10 ("index") 11 ("index") 12 ("index") 13 ("index") 14 ("index") 15 ("index")] -> w950
      frame "CO" {
      }
      frame "HC Cycle 1" {
      }
      frame "Air Cycle 1", Default {
      }
      frame "NO" {
      }
      frame "Air Bal" {
      }
      frame "HC Bal" {
      }
      frame "Air Cycle 2" {
      }
      frame "HC Cycle 2" {
      }
    }
    n404 = case shown="\"NO\", Default" "Graph 4 Box" {
      tunnel: [0 ("index") 1 ("index") 2 ("index") 3 ("index") 4 ("index") 5 ("index") 6 ("index") 7 ("index")] -> w947
      tunnel: [8 ("index") 9 ("index") 10 ("index") 11 ("index") 12 ("index") 13 ("index") 14 ("index") 15 ("index")] -> w948
      frame "CO" {
      }
      frame "HC Cycle 1" {
      }
      frame "Air Cycle 1" {
      }
      frame "NO", Default {
      }
      frame "Air Bal" {
      }
      frame "HC Bal" {
      }
      frame "Air Cycle 2" {
      }
      frame "HC Cycle 2" {
      }
    }
    n405 = call "Mexa_7170.vi"("String 1 In"=w931, "Connect"=w932, "connection ID 1 In"=w930, "error out 1 In"=w929, "connection ID 2 In"=w937, "error out 2 In"=w938, "Time In"=w940) -> ("Emissions"=w928:dbl[], "String 1 Out"=w933:string, "connection ID 1 Out"=w935:refnum<k5>, "error 1 out"=w934:errorcluster, "connection ID 2 Out"=w936:refnum<k16>, "Time Out"=w941:i16, "error 2 out"=w939:errorcluster)  [unwired: 2 in]
    "Mexa_One Emissions" <- w928
    n406 = Index Array(array=w959, index #1=w960, index #2=w967) -> (element #1=w962:dbl, element #2=w961:dbl)
    n407 = Index Array(array=w959, index #1=w951, index #2=w952) -> (element #1=w958:dbl, element #2=w957:dbl)
    n408 = Index Array(array=w959, index #1=w949, index #2=w950) -> (element #1=w956:dbl, element #2=w955:dbl)
    n409 = Index Array(array=w959, index #1=w947, index #2=w948) -> (element #1=w954:dbl, element #2=w953:dbl)
    n410 = Merge Signals(w962, w961) -> (→"MFC Graph 1":dynamicdata)
    n411 = Merge Signals(w958, w957) -> (→"MFC Graph 2":dynamicdata)
    n412 = Merge Signals(w956, w955) -> (→"MFC Graph 3":dynamicdata)
    n413 = Merge Signals(w954, w953) -> (→"MFC Graph 4":dynamicdata)
    n414 = call "MKS.vi"("IP Address"="192.168.254.2" ("IP_ADD [127.0.0.1]"), "Connect"="MKS 5Hz") -> ("Emissions"=w942:dbl[])  [unwired: 9 in]
    n415 = Build Array (concatenate)(w959, w928, w942) -> (w972:dbl[])
    n416 = for {
      tunnel: w972 -> [w1053] mode=indexing
      tunnel: [w1052] -> w975 mode=indexing
      n417 = Number To Fractional String(number=w1053, precision (6)=i16 3) -> (F-format string=w1052:string)  [unwired: 2 in]
    }
    n418 = shared-variable "RT CompactRIO Target 2\\Library 1.lvlib\\Analyser_Data"(w928) -> ()  [unwired: 1 in, 1 out]
    n419 = Get Date/Time In Seconds() -> (seconds since 1Jan1904=w978:timestamp)
    n420 = local read "File name"() -> (w982:string)
    n421 = Format Date/Time String(time format string (%c)="%d/%m/%y %H:%M:%S", seconds (now)=w978) -> (date/time string=w976:string)  [unwired: 1 in]
    n422 = Index Array(array=w942, index="HC Index") -> (element=→"MKS HC":dbl)
    n423 = Concatenate Strings(w982, "_MFC" ("string")) -> (w980:string)
    n424 = Build Array (concatenate)(w976, w975) -> (w974:string[])
    n425 = String To Path(string=w980) -> (path=w977:path)
    n426 = local read "Log?"() -> (w973:bool)
    n427 = case shown="True" w973 {
      tunnel: w977 -> [w1047 w1050]
      tunnel: [w1047 w1048] -> _
      tunnel: w974 -> [_ w1049]
      frame False {
      }
      frame True {
        n428 = call-poly <vilib>:"Write To Spreadsheet File.vi"("append to file? (new file:F)"=TRUE, "1D data"=w1049, "file path (dialog if empty)"=w1050) -> ("new file path (Not A Path if cancelled)"=w1048:path)  [unwired: 5 in]
      }
    }
    n429 = node-c288() -> ()  [unwired: 1 in, 1 out]
  }
  n430 = while {
    tunnel: w42 -> [w1061]
    tunnel: w26 -> [w1059]
    tunnel: w28 -> [w1058]
    tunnel: [FALSE ("stop 2")] -> w16
    stop <- w1062 stop-if-true
    n431 = Dequeue Element(queue=w1061) -> (element=w1060:T10)  [unwired: 2 in, 3 out]
    n432 = case shown="\"start test\"" w1060 {
      tunnel: w1059 -> [_ _ _ w1117 w1128 w1164 w1198 _ _ _ _ _ _ _ w1561 _ _ _ _ _ _ _ _]
      tunnel: w1058 -> [_ _ _ _ _ _ _ _ w1211 w1226 w1281 w1326 _ _ _ _ _ _ _ _ _ _ _]
      frame "main", Default {
        # "00 stop cmd\n01 Test Number\n02 Test Flow Rate\n03 Test Start Temperature\n04 Test Stop Temperature\n05 Furnace Ramp Rate\n06 Inlet Lambda\n07 Inlet O2\n08 Inlet Lambda Rich\n09 Inlet Lambda Lean\n10 Inlet Temperature\n11 NO SW"
        # "20"
        # "25"
        # "30"
        # "15"
        # "10"
        # "5"
        # "0"
        # "30"
        # "25"
        # "20"
        # "15"
        # "10"
        # "5"
        # "0"
        # "Output Cluster\n\n0 NOx Conc\n1 CO conc %\n2 HC conc %\n3 Bleed H2O \n4 Bleed CO2\n5 Bleed N2 \n6 lambda P\n7 lambda I\n8 lambda D\n9 purge duration\n10 Target furnace lambda\n11 HC reaction ct\n12 Full system\n13 Log interval\n14 MKS 1\n15 MKS 2"
        n433 = local read "output cluster"() -> (w1092:T2)
        n434 = Unbundle(w1092) -> ("NOx Concentration (ppm)"=w1079:T1, "CO concentration %"=w1078:T1, "HC concentration %"=w1077:T1, "Bleed H2O %"=w1076:T1, "Bleed CO2 %"=w1075:T1, "Bleed N2 %"=w1089:T1, "lambda P"=w1088:T1, "lambda I"=w1087:T1, "lambda D"=w1090:T1, "Purge duration (seconds)"=w1091:T1, "Target furnace lambda"=w1084:T1, "HC reaction constant"=w1083:T1, w1085:i16, "Log interval (HRS)"=→"Log interval (seconds)":T1, w1072:i16, w1071:i16, "Advanced Logging"=→"Advanced Logging":bool, "Cycle Length (Hours)"=w1070:T1, "Heat Load Control"=w1069:bool, w1067:T1[])
        n435 = local read "HC Theory (%)"() -> (w1063:T7)
        n436 = local read "Test Flow Rate(g/s)"() -> (w1103:T1)
        n437 = local read "Test number"() -> (w1108:u16)
        n438 = local read "CO Theory (%)"() -> (w1095:T7)
        n439 = local read "NO ppm Loff"() -> (w1094:T1)
        n440 = local read "Inlet O2 (%)"() -> (w1096:T1)
        n441 = local read "NO:CO Ratio"() -> (w1093:T1)
        n442 = local read "Connected"() -> (w1098:bool)
        n443 = Boolean To (0,1)(Boolean=w1069) -> (0, 1=w1068:i16)
        n444 = Boolean To (0,1)(Boolean=w1098) -> (0, 1=w1082:i16)
        n445 = Build Array (concatenate)("Stop Cmd", w1108, w1103, "Test Start Temperature (°C)", "Test Stop temperature (°C)", "Furnace Ramp Rate (°C/min)", w1096, w1095, w1063, "Inlet LAMBDA Lean", "Inlet Temperature (°C)", "NO ppm SW", w1094, w1093, "Temperature Limit (°C)", w1082, "Inlet temp Age", "Flow rate Age", w1079, w1078, w1077, w1076, w1075, w1089, w1088, w1087, w1090, w1091, w1084, w1083, w1085, w1070, w1068, w1067) -> (w1100:T1[])
        n446 = Not Equal To 0?(x=w1085) -> (x != 0?=→"Full System":bool)
        n447 = shared-variable "RT CompactRIO Target 2\\Library 1.lvlib\\Control Variables"(w1100) -> ()  [unwired: 1 in, 1 out]
        n448 = Not Equal To 0?(x=w1072) -> (x != 0?=w1073:bool)
        "Mexa One" <- w1073
        n449 = Not Equal To 0?(x=w1071) -> (x != 0?=w1066:bool)
        "MKS" <- w1066
        n450 = Or(x=w1073, y=w1066) -> (x .or. y?=→"Connected":bool)
      }
      frame "start test" {
        w1109 = FALSE
        n451 = property on="Pass" class="Bool (strict)"("Value"=w1109) -> ()  [unwired: 2 in, 2 out]
        n452 = property on="Fail" class="Bool (strict)"("Value"=w1109) -> ()  [unwired: 2 in, 2 out]
        n453 = local write "Pass"(w1109) -> ()
        n454 = local write "Fail"(w1109) -> ()
        n455 = shared-variable "RT CompactRIO Target 2\\Library 1.lvlib\\Enum 1"("Enum 1") -> ()  [unwired: 1 in, 1 out]
      }
      frame "clear table 1" {
        n456 = property on="Sub-Cycle Name" class="Str (strict)"("Value"="" ("Subcycle name")) -> ()  [unwired: 2 in, 2 out]
        n457 = local write "Sub-Cycle Pattern"(string[][] [["", "0", "", "", "", "", "", "", "", "", "", "", ""], ["", "", "", "", "", "", "", "", "", "", "", "", ""], ["", "", "", "", "", "", "", "", "", "", "", "", ""], ["", "", "", "", "", "", "", "", "", "", "", "", ""], ["", "", "", "", "", "", "", "", "", "", "", "", ""], ["", "", "", "", "", "", "", "", "", "", "", "", ""], ["", "", "", "", "", "", "", "", "", "", "", "", ""], ["", "", "", "", "", "", "", "", "", "", "", "", ""], ["", "", "", "", "", "", "", "", "", "", "", "", ""], ["", "", "", "", "", "", "", "", "", "", "", "", ""], ["", "", "", "", "", "", "", "", "", "", "", "", ""], ["", "", "", "", "", "", "", "", "", "", "", "", ""], ["", "", "", "", "", "", "", "", "", "", "", "", ""], ["", "", "", "", "", "", "", "", "", "", "", "", ""], ["", "", "", "", "", "", "", "", "", "", "", "", ""], ["", "", "", "", "", "", "", "", "", "", "", "", ""], ["", "", "", "", "", "", "", "", "", "", "", "", ""], ["", "", "", "", "", "", "", "", "", "", "", "", ""], ["", "", "", "", "", "", "", "", "", "", "", "", ""], ["", "", "", "", "", "", "", "", "", "", "", "", ""], ["", "", "", "", "", "", "", "", "", "", "", "", ""], ["", "", "", "", "", "", "", "", "", "", "", "", ""], ["", "", "", "", "", "", "", "", "", "", "", "", ""], ["", "", "", "", "", "", "", "", "", "", "", "", ""], ["", "", "", "", "", "", "", "", "", "", "", "", ""], ["", "", "", "", "", "", "", "", "", "", "", "", ""], ["", "", "", "", "", "", "", "", "", "", "", "", ""], ["", "", "", "", "", "", "", "", "", "", "", "", ""], ["", "", "", "", "", "", "", "", "", "", "", "", ""], ["", "", "", "", "", "", "", "", "", "", "", "", ""], ["", "", "", "", "", "", "", "", "", "", "", "", ""]]) -> ()
        n458 = local write "Flag1"(FALSE) -> ()
      }
      frame "update list 1" {
        n459 = String To Path(string=w1117) -> (path=w1116:path)
        n460 = List Folder(path=w1116, pattern="*.eyes") -> (filenames=w1115:string[])  [unwired: 2 in, 3 out]
        n461 = property on="Sub-Cycle List" class="LstBox (strict)"("Item Names"=w1115) -> ()  [unwired: 2 in, 2 out]
      }
      frame "save subc" {
        w1121 = ".eyes" ("string")
        n462 = local read "Sub-Cycle Name"() -> (w1120:T5)
        n463 = String To Path(string=w1128) -> (path=w1133:path)
        n464 = Equal?(x=w1120, y="") -> (x = y?=w1125:bool)
        n465 = List Folder(path=w1133, pattern="*.eyes" ("string")) -> (filenames=w1132:string[])  [unwired: 2 in, 3 out]
        n466 = Concatenate Strings(w1120, w1121) -> (w1119:string)
        n467 = Concatenate Strings(w1128, w1120, w1121) -> (w1134:string)
        n468 = Search 1D Array(1D array=w1132, element=w1119) -> (index of element=w1131:i32)  [unwired: 1 in]
        n469 = case shown="True" w1125 {
          tunnel: [TRUE FALSE] -> w1124
          frame False {
          }
          frame True {
            n470 = One Button Dialog(message="Insert file name!") -> ()  [unwired: 1 in, 1 out]
          }
        }
        n471 = String To Path(string=w1134) -> (path=w1127:path)
        n472 = Equal?(x=w1131, y=-1) -> (x = y?=w1129:bool)
        n473 = case shown="False" w1129 {
          selector: w1129 -> [_ w1140]
          tunnel: [w1138 w1140] -> w1123
          frame False {
            n474 = Two Button Dialog(message="A file with this name already exists!\nDo you want to overwrite?") -> (T button?=w1138:bool)  [unwired: 2 in]
          }
          frame True {
          }
        }
        n475 = And(x=w1123, y=w1124) -> (x .and. y?=w1122:bool)
        n476 = case shown="True" w1122 {
          tunnel: w1127 -> [_ w1145]
          frame False {
          }
          frame True {
            n477 = local read "Sub-Cycle Pattern"() -> (w1144:string[][])
            n478 = call "Table check.vi"("Input table"=w1144) -> ("Incomplete?"=w1142:bool, "Length"=w1143:i32)  [unwired: 9 in]
            n479 = case shown="False" w1142 {
              tunnel: w1144 -> [w1153 _]
              tunnel: w1145 -> [w1152 _]
              tunnel: w1143 -> [w1151 _]
              tunnel: string[] [] -> [w1150 _]
              frame False {
                n480 = for {
                  N: w1151 -> [_]
                  tunnel: w1153 -> [w1160]
                  shift-right: [w1157] -> w1149
                  shift-left: w1150 -> [w1158]
                  i -> [w1159]
                  n481 = Index Array(array=w1160, index (row)=w1159) -> (element=w1156:string[])  [unwired: 1 in]
                  n482 = Delete From Array(array=w1156, index=0) -> (array with subset deleted=w1155:string[])  [unwired: 1 in, 1 out]
                  n483 = Build Array (concatenate)(w1158, w1155) -> (w1157:string[])
                }
                n484 = Build Array (concatenate)("SubCycle Data File for EYECAT - do not modify", w1149) -> (w1147:string[])
                n485 = call-poly <vilib>:"Write To Spreadsheet File.vi"("1D data"=w1147, "file path (dialog if empty)"=w1152) -> ()  [unwired: 6 in, 1 out]
              }
              frame True {
                n486 = One Button Dialog(message="The table is incomplete!\nplease review and save again!") -> ()  [unwired: 1 in, 1 out]
              }
            }
            n487 = local write "Flag1"(FALSE) -> ()
          }
        }
      }
      frame "load subc" {
        n488 = local read "Flag1"() -> (w1165:bool)
        n489 = case shown="True" w1165 {
          tunnel: [w1192 w1194] -> w1163
          tunnel: w1164 -> [w1192 w1194]
          tunnel: [TRUE w1193] -> w1162
          frame False {
          }
          frame True {
            n490 = Two Button Dialog(message="The table has been modified.\nDo you want to continue?") -> (T button?=w1193:bool)  [unwired: 2 in]
          }
        }
        n491 = case shown="True" w1162 {
          tunnel: w1163 -> [_ w1169]
          frame False {
          }
          frame True {
            n492 = property on="Sub-Cycle List" class="LstBox (strict)"() -> ("Item Names"=w1181:string[])  [unwired: 2 in, 2 out]
            n493 = Index Array(array=w1181, index="Sub-Cycle List") -> (element=w1168:string)
            n494 = Concatenate Strings(w1169, w1168) -> (w1179:string)
            n495 = Search/Split String(string=w1168, search string/char (-)=".") -> (substring before match=w1166:string)  [unwired: 1 in, 2 out]
            n496 = local write "Sub-Cycle Name"(w1166) -> ()
            n497 = String To Path(string=w1179) -> (path=w1178:path)
            n498 = call-poly <vilib>:"Read From Spreadsheet File.vi"("file path (dialog if empty)"=w1178) -> ("first row"=w1174:string[])  [unwired: 6 in, 4 out]
            n499 = Delete From Array(array=w1174, length=1, index=0) -> (array with subset deleted=w1171:string[])  [unwired: 1 out]
            n500 = Array Size(array=w1171) -> (size(s)=w1177:i32)
            n501 = Divide(x=w1177, y=12) -> (x/y=w1170:dbl)
            n502 = for {
              N: w1170 -> [_]
              shift-right: [w1187] -> _
              shift-left: w1171 -> [w1190]
              tunnel: [w1186] -> w1175 mode=indexing
              i -> [w1185]
              n503 = Increment(x=w1185) -> (x+1=w1184:i32)
              n504 = Delete From Array(array=w1190, length=12, index=0) -> (deleted portion=w1182:string[], array with subset deleted=w1187:string[])
              n505 = Number To Decimal String(number=w1184) -> (decimal integer string=w1183:string)  [unwired: 1 in]
              n506 = Build Array (concatenate)(w1183, w1182) -> (w1186:string[])
            }
            n507 = local write "Sub-Cycle Pattern"(w1175) -> ()
          }
        }
      }
      frame "delete subc" {
        n508 = Two Button Dialog(message="This operation will permanently delete this file!\nDo you want to continue?") -> (T button?=w1197:bool)  [unwired: 2 in]
        n509 = case shown="True" w1197 {
          tunnel: w1198 -> [_ w1203]
          frame False {
          }
          frame True {
            n510 = local read "Sub-Cycle List"() -> (w1200:i32)
            n511 = property on="Sub-Cycle List" class="LstBox (strict)"() -> ("Item Names"=w1201:string[])  [unwired: 2 in, 2 out]
            n512 = Index Array(array=w1201, index=w1200) -> (element=w1205:string)
            n513 = Concatenate Strings(w1203, w1205) -> (w1204:string)
            n514 = local write "Flag1"(FALSE) -> ()
            n515 = String To Path(string=w1204) -> (path=w1202:path)
            n516 = Delete(path (use dialog)=w1202) -> ()  [unwired: 4 in, 3 out]
          }
        }
      }
      frame "clear table 2" {
        n517 = property on="Cycle Name" class="Str (strict)"("Value"="" ("Subcycle name")) -> ()  [unwired: 2 in, 2 out]
        n518 = local write "Flag 2"(FALSE) -> ()
        n519 = local write "Cycle Pattern"(string[][] [["", "", "", "", ""], ["", "", "", "", ""], ["", "", "", "", ""], ["", "", "", "", ""], ["", "", "", "", ""], ["", "", "", "", ""], ["", "", "", "", ""], ["", "", "", "", ""], ["", "", "", "", ""], ["", "", "", "", ""], ["", "", "", "", ""], ["", "", "", "", ""], ["", "", "", "", ""], ["", "", "", "", ""], ["", "", "", "", ""], ["", "", "", "", ""], ["", "", "", "", ""], ["", "", "", "", ""], ["", "", "", "", ""], ["", "", "", "", ""], ["", "", "", "", ""], ["", "", "", "", ""], ["", "", "", "", ""], ["", "", "", "", ""], ["", "", "", "", ""], ["", "", "", "", ""], ["", "", "", "", ""], ["", "", "", "", ""], ["", "", "", "", ""], ["", "", "", "", ""], ["", "", "", "", ""]]) -> ()
      }
      frame "update list 2" {
        n520 = String To Path(string=w1211) -> (path=w1212:path)
        n521 = List Folder(path=w1212, pattern="*.eyec") -> (filenames=w1210:string[])  [unwired: 2 in, 3 out]
        n522 = property on="Cycle List" class="LstBox (strict)"("Item Names"=w1210) -> ()  [unwired: 2 in, 2 out]
      }
      frame "save cycle" {
        w1213 = ".eyec" ("string")
        n523 = local read "Cycle Name"() -> (w1214:T5)
        n524 = String To Path(string=w1226) -> (path=w1227:path)
        n525 = List Folder(path=w1227, pattern="*.eyec" ("string")) -> (filenames=w1225:string[])  [unwired: 2 in, 3 out]
        n526 = Equal?(x=w1214, y="") -> (x = y?=w1220:bool)
        n527 = Concatenate Strings(w1214, w1213) -> (w1216:string)
        n528 = Search 1D Array(1D array=w1225, element=w1216) -> (index of element=w1224:i32)  [unwired: 1 in]
        n529 = Concatenate Strings(w1226, w1214, w1213) -> (w1229:string)
        n530 = case shown="True" w1220 {
          tunnel: [TRUE FALSE] -> w1218
          frame False {
          }
          frame True {
            n531 = One Button Dialog(message="Insert file name!") -> ()  [unwired: 1 in, 1 out]
          }
        }
        n532 = String To Path(string=w1229) -> (path=w1228:path)
        n533 = Equal?(x=w1224, y=-1) -> (x = y?=w1222:bool)
        n534 = case shown="False" w1222 {
          selector: w1222 -> [_ w1278]
          tunnel: [w1276 w1278] -> w1219
          frame False {
            n535 = Two Button Dialog(message="A file with this name already exists!\nDo you want to overwrite?") -> (T button?=w1276:bool)  [unwired: 2 in]
          }
          frame True {
          }
        }
        n536 = And(x=w1219, y=w1218) -> (x .and. y?=w1217:bool)
        n537 = case shown="True" w1217 {
          tunnel: w1228 -> [_ w1236]
          frame False {
          }
          frame True {
            n538 = local read "Cycle Pattern"() -> (w1235:string[][])
            n539 = call "Table check.vi"("Input table"=w1235) -> ("Incomplete?"=w1233:bool, "Length"=w1234:i32)  [unwired: 9 in]
            n540 = case shown="False" w1233 {
              tunnel: w1236 -> [w1245 _]
              tunnel: w1235 -> [w1244 _]
              tunnel: w1234 -> [w1237 _]
              frame False {
                n541 = Number To Decimal String(number=w1237) -> (decimal integer string=w1240:string)  [unwired: 1 in]
                n542 = for {
                  N: w1237 -> [_]
                  tunnel: w1244 -> [w1274]
                  shift-right: [w1262] -> w1241
                  shift-left: string[] [] -> [w1272]
                  i -> [w1273]
                  w1253 = 12 ("length")
                  n543 = Index Array(array=w1274, index (row)=w1273) -> (element=w1268:string[])  [unwired: 1 in]
                  n544 = Index Array(array=w1268, index=3) -> (element=w1258:string)
                  n545 = Index Array(array=w1268, index=1) -> (element=w1257:string)
                  n546 = Concatenate Strings("C:\\Setup Files\\Subcycles Folder\\", w1257) -> (w1269:string)
                  n547 = String To Path(string=w1269) -> (path=w1270:path)
                  n548 = call-poly <vilib>:"Read From Spreadsheet File.vi"("file path (dialog if empty)"=w1270) -> ("first row"=w1261:string[])  [unwired: 6 in, 4 out]
                  n549 = Delete From Array(array=w1261, length=1, index=0) -> (array with subset deleted=w1255:string[])  [unwired: 1 out]
                  n550 = String Length(string=w1255) -> (length=w1264:i32[])
                  n551 = Array Size(array=w1264) -> (size(s)=w1256:i32)
                  n552 = Divide(x=w1256, y=w1253) -> (x/y=w1254:dbl)
                  n553 = Decrement(x=w1254) -> (x-1=w1246:dbl)
                  n554 = Multiply(x=w1253, y=w1246) -> (x*y=w1252:dbl)
                  n555 = Number To Decimal String(number=w1246) -> (decimal integer string=w1263:string)  [unwired: 1 in]
                  n556 = Delete From Array(array=w1255, length=12, index=w1252) -> (deleted portion=w1249:string[], array with subset deleted=w1250:string[])
                  n557 = Index Array(array=w1249, index=0) -> (element=w1247:string)
                  n558 = Build Array (concatenate)(w1257, w1258, w1263, w1247, w1250) -> (w1267:string[])
                  n559 = Build Array (concatenate)(w1272, w1267) -> (w1262:string[])
                }
                n560 = local write "Flag 2"(FALSE) -> ()
                n561 = Build Array (concatenate)("Cycle Data File for EYECAT - do not modify", w1240, w1241) -> (w1242:string[])
                n562 = call-poly <vilib>:"Write To Spreadsheet File.vi"("1D data"=w1242, "file path (dialog if empty)"=w1245) -> ()  [unwired: 6 in, 1 out]
              }
              frame True {
                n563 = One Button Dialog(message="The table is incomplete!\nplease review and save again!") -> ()  [unwired: 1 in, 1 out]
              }
            }
          }
        }
      }
      frame "load cycle" {
        n564 = local read "Flag 2"() -> (w1282:bool)
        n565 = case shown="True" w1282 {
          tunnel: [w1321 w1323] -> w1279
          tunnel: w1281 -> [w1321 w1323]
          tunnel: [TRUE ("T button?") w1322] -> w1280
          frame False {
          }
          frame True {
            n566 = Two Button Dialog(message="The table has been modified.\nDo you want to continue?") -> (T button?=w1322:bool)  [unwired: 2 in]
          }
        }
        n567 = case shown="True" w1280 {
          tunnel: w1279 -> [_ w1285]
          frame False {
          }
          frame True {
            n568 = property on="Cycle List" class="LstBox (strict)"() -> ("Item Names"=w1301:string[])  [unwired: 2 in, 2 out]
            n569 = Index Array(array=w1301, index="Cycle List") -> (element=w1287:string)
            n570 = Concatenate Strings(w1285, w1287) -> (w1300:string)
            n571 = Search/Split String(string=w1287, search string/char (-)=".") -> (substring before match=w1286:string)  [unwired: 1 in, 2 out]
            n572 = String To Path(string=w1300) -> (path=w1299:path)
            n573 = local write "Cycle Name"(w1286) -> ()
            n574 = call-poly <vilib>:"Read From Spreadsheet File.vi"("file path (dialog if empty)"=w1299) -> ("first row"=w1283:string[])  [unwired: 6 in, 4 out]
            n575 = Delete From Array(array=w1283, length=2, index=0) -> (array with subset deleted=w1284:string[])  [unwired: 1 out]
            n576 = Index Array(array=w1283, index=1) -> (element=w1298:string)
            n577 = Decimal String To Number(string=w1298) -> (number=w1297:i32)  [unwired: 2 in, 1 out]
            n578 = for {
              N: w1297 -> [_]
              tunnel: w1284 -> [w1319]
              tunnel: [w1314] -> w1292 mode=indexing
              shift-right: [w1304] -> _
              shift-left: 0 ("x") -> [w1305]
              i -> [w1318]
              w1315 = ""
              n579 = Increment(x=w1305) -> (x+1=w1303:i32)
              n580 = Increment(x=w1303) -> (x+1=w1311:i32)
              n581 = Increment(x=w1318) -> (x+1=w1313:i32)
              n582 = Number To Decimal String(number=w1313) -> (decimal integer string=w1312:string)  [unwired: 1 in]
              n583 = Index Array(array=w1319, index #1=w1305, index #2=w1303, index #3=w1311) -> (element #1=w1317:string, element #2=w1316:string, element #3=w1310:string)
              n584 = Build Array(w1312, w1317, w1315, w1316, w1315) -> (w1314:string[])
              n585 = Decimal String To Number(string=w1310) -> (number=w1309:i32)  [unwired: 2 in, 1 out]
              n586 = Multiply(x=w1309, y=12 ("x")) -> (x*y=w1307:i32)
              n587 = Compound Arithmetic op=ADD(w1307, 4, w1305) -> (w1304:i32)
            }
            n588 = Insert Into Array(array=string[][] [["", "", "", "", ""], ["", "", "", "", ""], ["", "", "", "", ""], ["", "", "", "", ""], ["", "", "", "", ""], ["", "", "", "", ""], ["", "", "", "", ""], ["", "", "", "", ""], ["", "", "", "", ""], ["", "", "", "", ""], ["", "", "", "", ""], ["", "", "", "", ""], ["", "", "", "", ""], ["", "", "", "", ""], ["", "", "", "", ""], ["", "", "", "", ""], ["", "", "", "", ""], ["", "", "", "", ""], ["", "", "", "", ""], ["", "", "", "", ""], ["", "", "", "", ""], ["", "", "", "", ""], ["", "", "", "", ""], ["", "", "", "", ""], ["", "", "", "", ""], ["", "", "", "", ""], ["", "", "", "", ""], ["", "", "", "", ""], ["", "", "", "", ""], ["", "", "", "", ""], ["", "", "", "", ""]], index (row)=0, new element=w1292) -> (w1291:string[][])  [unwired: 1 in]
            n589 = local write "Cycle Pattern"(w1291) -> ()
          }
        }
      }
      frame "delete cycle" {
        n590 = Two Button Dialog(message="This operation will permanently delete this file!\nDo you want to continue?") -> (T button?=w1327:bool)  [unwired: 2 in]
        n591 = case shown="True" w1327 {
          tunnel: w1326 -> [_ w1332]
          frame False {
          }
          frame True {
            n592 = local read "Cycle List"() -> (w1333:i32)
            n593 = property on="Cycle List" class="LstBox (strict)"() -> ("Item Names"=w1334:string[])  [unwired: 2 in, 2 out]
            n594 = Index Array(array=w1334, index=w1333) -> (element=w1331:string)
            n595 = Concatenate Strings(w1332, w1331) -> (w1330:string)
            n596 = String To Path(string=w1330) -> (path=w1329:path)
            n597 = Delete(path (use dialog)=w1329) -> ()  [unwired: 4 in, 3 out]
            n598 = local write "Flag 2"(FALSE) -> ()
          }
        }
      }
      frame "calc HC CO" {
        n599 = local read "Sub-Cycle Pattern"() -> (w1351:string[][])
        n600 = Index Array(array=w1351, index (col) #1=3 ("disabled index (col)"), index (col) #2=4 ("index (col)"), index (col) #3=11 ("index (col)")) -> (element #1=w1341:string[], element #2=w1348:string[], element #3=w1335:string[])  [unwired: 3 in]
        n601 = Array Size(array=w1341) -> (size(s)=w1339:i32)
        n602 = Search 1D Array(1D array=w1341, element="") -> (index of element=w1338:i32)  [unwired: 1 in]
        n603 = Equal?(x=w1338, y=-1) -> (x = y?=w1340:bool)
        n604 = Select(t=w1339, s=w1340, f=w1338) -> (s? t:f=w1337:i32)
        n605 = for {
          N: w1337 -> [_]
          tunnel: [w1362] -> w1345 mode=indexing
          tunnel: [w1361] -> w1344 mode=indexing
          tunnel: w1341 -> [w1360] mode=indexing
          tunnel: w1348 -> [w1359] mode=indexing
          tunnel: w1335 -> [w1358] mode=indexing
          w1357 = ""
          n606 = Not Equal?(x=w1360, y=w1357) -> (x != y?=w1356:bool)
          n607 = Not Equal?(x=w1359, y=w1357) -> (x != y?=w1355:bool)
          n608 = Not Equal?(x=w1358, y=w1357) -> (x != y?=w1354:bool)
          n609 = Compound Arithmetic op=AND(w1356, w1355, w1354) -> (w1353:bool)
          n610 = case shown="True" w1353 {
            tunnel: w1360 -> [_ w1391]
            tunnel: w1359 -> [_ w1390]
            tunnel: [w1363 w1387] -> w1361
            tunnel: [w1363 w1386] -> w1362
            tunnel: w1358 -> [_ w1364]
            frame False {
              w1363 = ""
            }
            frame True {
              # "O2Eq"
              n611 = Fract/Exp String To Number(string=w1364) -> (number=w1365:dbl)  [unwired: 3 in, 1 out]
              n612 = Fract/Exp String To Number(string=w1391) -> (number=w1372:dbl)  [unwired: 3 in, 1 out]
              n613 = Fract/Exp String To Number(string=w1390) -> (number=w1368:dbl)  [unwired: 3 in, 1 out]
              n614 = Decrement(x=w1372) -> (x-1=w1373:dbl)
              n615 = Divide(x=w1365, y=20000.0) -> (x/y=w1366:dbl)
              n616 = Multiply(x=4.76, y=w1372) -> (x*y=w1377:dbl)
              n617 = Multiply(x=w1373, y=100.0) -> (x*y=w1375:dbl)
              n618 = Add(x=w1368, y=w1366) -> (x+y=w1369:dbl)
              n619 = Add(x=0.33, y=w1377) -> (x+y=w1379:dbl)
              n620 = Divide(x=w1375, y=w1379) -> (x/y=w1380:dbl)
              n621 = Subtract(x=w1369, y=w1380) -> (x-y=w1382:dbl)
              n622 = Multiply(x=w1382, y=2.0) -> (x*y=w1370:dbl)
              n623 = Divide(x=w1382, y=5.0) -> (x/y=w1371:dbl)
              n624 = Number To Fractional String(number=w1371, width (-)=i16 6, precision (6)=i16 3) -> (F-format string=w1386:string)  [unwired: 1 in]
              n625 = Number To Fractional String(number=w1370, width (-)=i16 6, precision (6)=i16 2) -> (F-format string=w1387:string)  [unwired: 1 in]
            }
          }
        }
        n626 = Replace Array Subset(array=w1351, new element #1=w1345, index (col) #1=5 ("disabled index (col)"), new element #2=w1344, index (col) #2=6 ("disabled index (col)")) -> (w1349:string[][])  [unwired: 2 in]
        n627 = local write "Sub-Cycle Pattern"(w1349) -> ()
      }
      frame "Total time calc" {
        w1406 = i16 2 ("width (-)")
        w1413 = ":"
        n628 = local read "Cycle Pattern"() -> (w1420:string[][])
        n629 = Index Array(array=w1420, index (col)=4 ("disabled index (col)")) -> (element=w1393:string[])  [unwired: 1 in]
        n630 = Array Size(array=w1393) -> (size(s)=w1395:i32)
        n631 = Search 1D Array(1D array=w1393, element="") -> (index of element=w1394:i32)  [unwired: 1 in]
        n632 = Equal?(x=w1394, y=-1) -> (x = y?=w1396:bool)
        n633 = Select(t=w1395, s=w1396, f=w1394) -> (s? t:f=w1392:i32)
        n634 = for {
          N: w1392 -> [_]
          tunnel: w1393 -> [w1428] mode=indexing
          shift-right: [w1430] -> w1416
          shift-left: 0 -> [w1431]
          n635 = xnode "Match Regular Expression"("input string"=w1428, "regular expression"=":" ("search string/char (-)")) -> ("before match"=w1427:string, "after match"=w1424:string)  [unwired: 4 in, 3 out]
          n636 = Decimal String To Number(string=w1427) -> (number=w1426:i32)  [unwired: 2 in, 1 out]
          n637 = Decimal String To Number(string=w1424) -> (number=w1423:i32)  [unwired: 2 in, 1 out]
          n638 = Multiply(x=w1426, y=60) -> (x*y=w1422:i32)
          n639 = Add(x=w1422, y=w1423) -> (x+y=w1421:i32)
          n640 = Add(x=w1421, y=w1431) -> (x+y=w1430:i32)
        }
        n641 = local read "Total Number of Cycles"() -> (w1417:T1)
        n642 = Multiply(x=w1416, y=w1417) -> (x*y=w1412:T1)
        n643 = Quotient & Remainder(x=w1412, y=3600.0) -> (x-y*floor(x/y)=w1399:T1, floor(x/y)=w1409:T1)
        n644 = Quotient & Remainder(x=w1399, y=60.0) -> (x-y*floor(x/y)=w1407:T1, floor(x/y)=w1408:T1)
        n645 = Number To Decimal String(number=w1409) -> (decimal integer string=w1414:string)  [unwired: 1 in]
        n646 = Number To Decimal String(number=w1408, width (-)=w1406) -> (decimal integer string=w1410:string)
        n647 = Number To Decimal String(number=w1407, width (-)=w1406) -> (decimal integer string=w1405:string)
        n648 = Concatenate Strings(w1414, w1413, w1410, w1413, w1405) -> (w1404:string)
        n649 = call <vilib>:"Search and Replace Pattern.vi"("string"=w1404, "regular expression (\"\")"=" " ("replace string (\"\")"), "replace string (\"\")"="0" ("replace string (\"\")"), "replace all? (F)"=TRUE) -> ("result string"=→"Total Test Duration (hrs)":string)  [unwired: 1 in, 1 out]
      }
      frame "update Cycle pattern " {
        n650 = local read "Cycle Pattern"() -> (w1559:string[][])
        n651 = Index Array(array=w1559, index (col)=1 ("disabled index (col)")) -> (element=w1544:string[])  [unwired: 1 in]
        n652 = String To Path(string=w1561) -> (path=w1562:path)
        n653 = Array Size(array=w1544) -> (size(s)=w1547:i32)
        n654 = Search 1D Array(1D array=w1544, element="") -> (index of element=w1546:i32)  [unwired: 1 in]
        n655 = List Folder(path=w1562, pattern="*.eyes") -> (filenames=w1560:string[])  [unwired: 2 in, 3 out]
        n656 = Equal?(x=w1546, y=-1) -> (x = y?=w1548:bool)
        n657 = Select(t=w1547, s=w1548, f=w1546) -> (s? t:f=w1545:i32)
        n658 = for {
          N: w1545 -> [_]
          tunnel: w1559 -> [w1578] mode=indexing
          tunnel: w1561 -> [w1571]
          tunnel: [w1573] -> w1554 mode=indexing
          tunnel: [w1575] -> w1558 mode=indexing
          tunnel: [w1572] -> w1555 mode=indexing
          tunnel: w1560 -> [w1570]
          tunnel: [w1565] -> w1551 mode=indexing
          n659 = Index Array(array=w1578, index #1=1 ("index"), index #2=3 ("index")) -> (element #1=w1569:string, element #2=w1574:string)
          n660 = Search 1D Array(1D array=w1570, element=w1569) -> (index of element=w1568:i32)  [unwired: 1 in]
          n661 = Not Equal?(x=w1568, y=-1) -> (x != y?=w1566:bool)
          n662 = case shown="True" w1566 {
            tunnel: [w1582 w1596] -> w1575
            tunnel: w1574 -> [_ w1592]
            tunnel: [w1582 w1590] -> w1573
            tunnel: [w1582 w1589] -> w1572
            tunnel: w1571 -> [_ w1588]
            tunnel: w1569 -> [w1581 w1587]
            tunnel: [w1580 w1587] -> w1565
            frame False {
              w1582 = "N/A" ("String")
              n663 = Concatenate Strings(w1581, " - File NOT AVAILABLE !!!" ("string")) -> (w1580:string)
            }
            frame True {
              w1600 = i16 2 ("width (-)")
              n664 = Concatenate Strings(w1588, w1587) -> (w1618:string)
              n665 = String To Path(string=w1618) -> (path=w1617:path)
              n666 = call <vilib>:"Search and Replace Pattern.vi"("string"=w1592, "regular expression (\"\")"="[a-x ]" ("format string"), "replace string (\"\")"="", "replace all? (F)"=TRUE) -> ("result string"=w1589:string)  [unwired: 1 in, 1 out]
              n667 = call-poly <vilib>:"Read From Spreadsheet File.vi"("file path (dialog if empty)"=w1617) -> ("first row"=w1586:string[])  [unwired: 6 in, 4 out]
              n668 = Delete From Array(array=w1586, length=1, index=0) -> (array with subset deleted=w1585:string[])  [unwired: 1 out]
              n669 = Array Size(array=w1585) -> (size(s)=w1616:i32)
              n670 = Equal?(x=w1589, y="") -> (x = y?=w1604:bool)
              n671 = Subtract(x=w1616, y=12) -> (x-y=w1614:i32)
              n672 = Select(t="0", s=w1604, f=w1589) -> (s? t:f=w1603:string)
              n673 = Index Array(array=w1585, index=w1614) -> (element=w1590:string)
              n674 = Decimal String To Number(string=w1603) -> (number=w1613:i32)  [unwired: 2 in, 1 out]
              n675 = Decimal String To Number(string=w1590) -> (number=w1612:i32)  [unwired: 2 in, 1 out]
              n676 = Multiply(x=w1613, y=w1612) -> (x*y=w1611:i32)
              n677 = Quotient & Remainder(x=w1611, y=60) -> (x-y*floor(x/y)=w1609:i32, floor(x/y)=w1608:i32)
              n678 = Number To Decimal String(number=w1609, width (-)=w1600) -> (decimal integer string=w1606:string)
              n679 = Number To Decimal String(number=w1608, width (-)=w1600) -> (decimal integer string=w1605:string)
              n680 = Concatenate Strings(w1605, ":", w1606) -> (w1599:string)
              n681 = call <vilib>:"Search and Replace Pattern.vi"("string"=w1599, "regular expression (\"\")"=" " ("replace string (\"\")"), "replace string (\"\")"="0" ("replace string (\"\")"), "replace all? (F)"=TRUE) -> ("result string"=w1596:string)  [unwired: 1 in, 1 out]
            }
          }
        }
        n682 = Replace Array Subset(array=w1559, new element #1=w1551, index (col) #1=1 ("disabled index (col)"), new element #2=w1554, index (col) #2=2 ("disabled index (col)"), new element #3=w1555, index (col) #3=3 ("disabled index (col)"), new element #4=w1558, index (col) #4=4 ("disabled index (col)")) -> (w1563:string[][])  [unwired: 4 in]
        n683 = local write "Cycle Pattern"(w1563) -> ()
      }
      frame "load cycle name" {
        n684 = property on="Cycle Pattern" class="Tbl (strict)"() -> ("EditPos"=w1624:T3)  [unwired: 2 in, 2 out]
        n685 = Unbundle By Name(w1624) -> ("Row"=w1622:i32, "Column"=w1621:i32)
        n686 = local read "Cycle Pattern"() -> (w1620:string[][])
        n687 = call "SubCycles list.vi"() -> ("Subcycle name"=w1623:string)  [unwired: 10 in, 1 out]
        n688 = Replace Array Subset(array=w1620, new element=w1623, index (row)=w1622, index (col)=w1621) -> (w1619:string[][])
        n689 = local write "Cycle Pattern"(w1619) -> ()
      }
      frame "load test array" {
        n690 = local read "Total Test Duration (hrs)"() -> (w1632:T8)
        n691 = local read "Cycle Name"() -> (w1628:T5)
        n692 = Equal?(x=w1628, y="") -> (x = y?=w1627:bool)
        n693 = Not Equal?(x=w1632, y="0:00:00") -> (x != y?=w1626:bool)
        n694 = Or(x=w1626, y=w1627) -> (x .or. y?=w1625:bool)
        n695 = case shown="True" w1625 {
          selector: w1625 -> [w1633 _]
          tunnel: [FALSE TRUE] -> w1630
          frame False {
            n696 = case shown="False" w1633 {
              frame False {
                n697 = One Button Dialog(message="Incomplete Data!\nReview the cycle pattern!") -> ()  [unwired: 1 in, 1 out]
              }
              frame True {
              }
            }
          }
          frame True {
            w1639 = 0.0 ("default (0 I32)")
            n698 = local read "Cycle Name"() -> (w1654:T5)
            n699 = Concatenate Strings("C:\\Setup Files\\Cycles Folder\\", w1654, ".eyec" ("string")) -> (w1652:string)
            n700 = String To Path(string=w1652) -> (path=w1653:path)
            n701 = local read "Total Number of Cycles"() -> (w1650:T1)
            n702 = call-poly <vilib>:"Read From Spreadsheet File.vi"("file path (dialog if empty)"=w1653) -> ("first row"=w1636:string[])  [unwired: 6 in, 4 out]
            n703 = call "Remove names.vi"("Array in"=w1636) -> ("Array out"=w1645:string[])  [unwired: 10 in]
            n704 = Index Array(array=w1636, index #1=14 ("index"), index #2=15 ("index")) -> (element #1=w1641:string, element #2=w1637:string)
            n705 = Number To Decimal String(number="Ageing Gas") -> (decimal integer string=w1649:string)  [unwired: 1 in]
            n706 = Number To Decimal String(number=w1650) -> (decimal integer string=w1648:string)  [unwired: 1 in]
            n707 = Decimal String To Number(string=w1637, default (0L)=w1639) -> (number=w1638:dbl)  [unwired: 1 in, 1 out]
            n708 = Decimal String To Number(string=w1641, default (0L)=w1639) -> (number=w1640:dbl)  [unwired: 1 in, 1 out]
            n709 = property on="Inlet temp Age" class="DigNum (strict)"("Value"=w1640) -> ()  [unwired: 2 in, 2 out]
            n710 = property on="Flow rate Age" class="DigNum (strict)"("Value"=w1638) -> ()  [unwired: 2 in, 2 out]
            n711 = Build Array (concatenate)(w1649, w1648, w1645) -> (w1644:string[])
            n712 = shared-variable "RT CompactRIO Target 2\\Library 1.lvlib\\Ageing Variables"(w1644) -> ()  [unwired: 1 in, 1 out]
          }
        }
        "Test Compiled" <- w1630
      }
      frame "convert to num" {
        n713 = local read "EditPos Subc"() -> (w1659:T3)
        n714 = Unbundle By Name(w1659) -> ("Row"=w1660:i32, "Column"=w1657:i32)
        n715 = Equal?(x=w1657, y=7) -> (x = y?=w1656:bool)
        n716 = case shown="False" w1656 {
          tunnel: w1660 -> [_ w1665]
          tunnel: w1657 -> [_ w1663]
          tunnel: w1659 -> [_ _]
          frame True {
          }
          frame False {
            n717 = local read "Sub-Cycle Pattern"() -> (w1662:string[][])
            n718 = call "Conv to num.vi"("Column"=w1663, "Row"=w1665, "Array"=w1662) -> ("result string"=w1664:string)  [unwired: 8 in]
            n719 = Replace Array Subset(array=w1662, new element=w1664, index (row)=w1665, index (col)=w1663) -> (w1661:string[][])
            n720 = local write "Sub-Cycle Pattern"(w1661) -> ()
          }
        }
      }
      frame "check scycle name" {
        n721 = local read "Sub-Cycle Name"() -> (w1666:T5)
        n722 = call <vilib>:"Search and Replace Pattern.vi"("string"=w1666, "regular expression (\"\")"="[^0-9a-zA-Z ]" ("format string"), "replace string (\"\")"="", "replace all? (F)"=TRUE) -> ("result string"=w1672:string)  [unwired: 1 in, 1 out]
        n723 = Not Equal?(x=w1672, y=w1666) -> (x != y?=w1671:bool)
        n724 = case shown="False" w1671 {
          tunnel: w1672 -> [w1673 w1674]
          tunnel: [w1673 w1674] -> w1667
          frame False {
          }
          frame True {
            n725 = One Button Dialog(message="Unsuitable character for the file name!") -> ()  [unwired: 1 in, 1 out]
          }
        }
        n726 = local write "Sub-Cycle Name"(w1667) -> ()
      }
      frame "check cycle name" {
        n727 = local read "Cycle Name"() -> (w1676:T5)
        n728 = call <vilib>:"Search and Replace Pattern.vi"("string"=w1676, "regular expression (\"\")"="[^0-9a-zA-Z ]" ("format string"), "replace string (\"\")"="", "replace all? (F)"=TRUE) -> ("result string"=w1682:string)  [unwired: 1 in, 1 out]
        n729 = Not Equal?(x=w1682, y=w1676) -> (x != y?=w1681:bool)
        n730 = case shown="False" w1681 {
          tunnel: w1682 -> [w1683 w1684]
          tunnel: [w1683 w1684] -> w1677
          frame False {
          }
          frame True {
            n731 = One Button Dialog(message="Unsuitable character for the file name!") -> ()  [unwired: 1 in, 1 out]
          }
        }
        n732 = local write "Cycle Name"(w1677) -> ()
      }
      frame "Multigas connect" {
        # "add here logic to verify the user requirements and the machine state\n0 - not connected\n1 - MKS1 & Ext An Up\n2 - MKS2 & Ext An Dn\n3 - MKS 1 & 2  & Ext An Up & Dn"
        n733 = flat-sequence {
          frame #0 {
            "Connected?" <- TRUE
          }
        }
      }
      frame "Multigas disconnect" {
      }
      frame "Leak Test" {
        n734 = call "Press_Test.vi"() -> ("Reset Button"=w1687:bool)  [unwired: 11 in]
        n735 = local write "Leak Test"(w1687) -> ()
      }
    }
    n736 = local read "stop 2"() -> (w1062:bool)
  }
  n737 = node-c288(w7) -> ()  [unwired: 1 out]
  n738 = local write "stop 2"(w16) -> ()
  n739 = node-c288(w14) -> ()  [unwired: 1 out]
  "Table" <- string[][] [] ("Table")
